vi "commander3.vi"() -> ()   [LabVIEW 2012]
uses:
  G_SEN.vi
  G_VEH.vi
  G_LCM.vi
  G_PATH.vi
  G_NAV.vi
  G_DATA.vi
  <vilib>/Analysis/Matrix/Datatypes/RealMatrix.ctl
  <vilib>/Analysis/Matrix/NI_Matrix.lvlib
panel:
  in  "x 2":dbl
  in  "mobileye":bool
  out "LCM Recv Data":string
  out "GPS DATA 2":T1={"type"="None", "x_lcc"=-59.06772232055664, "y_lcc"=-26.082616806030273, "latdev"=0.0, "londev"=0.0, "sats"=0, "gps_l1_ranges"=0, "gps_l1_mask_ranges"=0, "gps_l2_mask_ranges"=0, "Heading"=89.78975677490234, "lon"=0.0, "lat"=0.0, "time"="None", "hgps"=89.78975677490234, "lag"=89.78975677490234, "MAP"="None"} {"lag" format="%#_5g"; "hgps" format="%#_5g"; "lat" format="%#_11g"; "lon" format="%#_11g"; "Heading" format="%#_5g"; "latdev" format="%#_4g"; "londev" format="%#_4g"}
  in  "LCM":bool
  in  "obs":bool
  in  "x":dbl
  in  "log":bool
  in  "y":dbl min=-1.0 max=10.0 step=0.1
  out "timmer 2":u32
  out "timmer":u32
  out "Speed limit":dbl=8.0
  out "collision":bool
  out "Mission":i32=9
  in  "Load WPT":bool
  in  "Max. Vel.":dbl=20.0
  in  "RESET PATH":bool
  out "col":i16(graph)
  out "stop":bool
  in  "Reverse":bool
  in  "STOP":bool
  out "Waveform Chart 4":cluster{"auto":i16, "run":i16}(graph)={"auto"=1, "run"=0}
  out "Waveform Chart 3":T2(graph)={"Steer_input"=10.50986504720403, "Steer_output"=3.6, "handle"=10.50986504720403}
  out "Waveform Chart 2":T3(graph)={"VS_des"=4.606086314285715, "VS_can"=8.738, "VS_des"=5.0237113142857135}
  out "Heading":cluster{"Heading":dbl, "hgps":dbl}(graph)={"Heading"=269.76568785604456, "hgps"=270.2149981902155}
  out "XY Graph 2":cluster{"Y":dbl[], "Y":dbl[]}[](graph)=[{"Y"=[-241.57278442382812], "Y"=[-497.6172790527344]}, {"Y"=array[297 elements], "Y"=array[297 elements]}, {"Y"=array[297 elements], "Y"=array[297 elements]}, {"Y"=[-96.81030887093378], "Y"=[-438.1146154201037]}]
  out "Gauge":cluster{dbl, dbl, dbl}(knob)={4.606086314285715, 8.738, 5.0237113142857135} scale=-20.0..140.0
  out "Meter":cluster{dbl, dbl, dbl}(knob)={10.50986504720403, 3.6, 10.50986504720403} scale=-550.0..550.0
  out "XY Graph":cluster{"Y":dbl[], "Y":dbl[]}[](graph)=[{"Y"=[0.0], "Y"=[1000.0]}, {"Y"=[], "Y"=[]}, {"Y"=[], "Y"=[]}, {"Y"=[55.79381017995934], "Y"=[-143.41137512848826]}, {"Y"=[1.8243630881955273], "Y"=[-0.6091599202647308]}, {"Y"=[60.825233010671326, 56.37330625127248, 55.349089235151354, 59.801015994550255, 60.825233010671326], "Y"=[-144.72018116547483, -142.44414335187238, -144.44751039360185, -146.72354820720435, -144.72018116547483]}, {"Y"=[0.0, 2.210107140854234e-06, 8.840428449730098e-06, 1.9890964154001267e-05, 3.536171391260723e-05, 5.5252677611861145e-05, 7.956385525176302e-05, 0.00010829524660493917, 0.00014144685155770276, 0.0001790186695416196, 0.00022101070067037654, 0.00026742294460291305, 0.00031825540077079495, 0.00037350806894664856, 0.0004331809489031002, 0.0004972740399580289, 0.0005657873416566872, 0.0006387208537717015, 0.0007160745756209508, 0.0007978485066360008, 0.0008840426462484174, 0.0009746569938897665, 0.0010696915488779268, 0.0011691463105307776, 0.0012730212781661976, 0.001381316451102066, 0.0014940318285425747, 0.0016111674095782291, 0.0017327231935269083, 0.0018586991794791174, 0.001989095366525362, 0.00212391175364246, 0.002263148340148291, 0.0024068051247922995, 0.002554882106551304, 0.0027073792846294964, 0.002864296657776322, 0.003025634224741225, 0.003191391984614711, 0.0033615699362599116, 0.003536168078198898, 0.0037151864094084885, 0.003898624928524441, 0.004086483634296201, 0.004278762525359525, 0.004475461600350172, 0.0046765808579039, 0.004882120296656467, 0.0050920799150162566, 0.00530645971150534, 0.005525259684645789, 0.005748479832959674, 0.005976120154741693, 0.006208180648513917, 0.006444661312457356, 0.006685562145094082, 0.006930883144491418, 0.007180624309171435, 0.007434785636974084, 0.007693367126535122, 0.007956368775921874, 0.008223790583087975, 0.008495632546100751, 0.008771894663368585, 0.009052576932504053, 0.00933767935191554, 0.009627201919329309, 0.009921144632812684, 0.010219507490205615, 0.010522290489461739, 0.010829493628421005, 0.011141116904923365, 0.011457160316581394, 0.011777623861462416, 0.012102507536951634, 0.012431811341116372, 0.012765535271228146, 0.013103679325240591, 0.0134462435006526, 0.013793227794963059, 0.014144632205784546, 0.014500456730615952, 0.014860701366956164, 0.015225366112190386, 0.015594450963703821, 0.015967955919109045, 0.0163458809754502, 0.016728226130226176, 0.017114991380822175, 0.017506176724168654, 0.0179017821577645, 0.018301807678767545, 0.018706253284335617, 0.019115118971512857, 0.019528404737457095, 0.01994611057932616, 0.02036823649393682, 0.02079478247856059, 0.021225748530014243, 0.02166113464522823, 0.022100940821246695], "Y"=[0.0, 0.05249999993797367, 0.10499999950378934, 0.15749999832528905, 0.2099999960303148, 0.26249999224670867, 0.31499998660231265, 0.3674999787249688, 0.41999996824251923, 0.472499954782806, 0.5249999379736712, 0.577499917442957, 0.6299998928185055, 0.682499863728159, 0.7349998297997596, 0.7874997906611497, 0.8399997459401715, 0.8924996952646672, 0.9449996382624795, 0.9974995745614504, 1.0499995037894228, 1.1024994255742389, 1.1549993395437415, 1.2074992453257731, 1.2599991425481762, 1.3124990308387938, 1.3649989098254687, 1.4174987791360436, 1.4699986383983614, 1.5224984872402658, 1.574998325289599, 1.6274981521742047, 1.6799979675219257, 1.7324977709606055, 1.784997562118088, 1.837497340622216, 1.8899971061008334, 1.9424968581817836, 1.994996596492911, 2.047496320662059, 2.099996030317072, 2.152495725085793, 2.204995404596067, 2.2574950684757384, 2.309994716352652, 2.3624943478546507, 2.414993962609581, 2.467493560245286, 2.519993140389611, 2.5724927026704023, 2.6249922467155042, 2.6774917721527607, 2.7299912786100196, 2.7824907657151243, 2.834990233095921, 2.887489680380256, 2.939989107195975, 2.9924885131709242, 3.0449878979329497, 3.0974872611098974, 3.1499866023296144, 3.2024859212199472, 3.2549852174087435, 3.3074844905238483, 3.3599837401931105, 3.412482966044377, 3.464982167705495, 3.5174813448043127, 3.5699804969686775, 3.6224796238264374, 3.6749787250054404, 3.7274778001335362, 3.7799768488385714, 3.8324758707483966, 3.884974865490859, 3.9374738326938097, 3.989972771985096, 4.042471682992569, 4.094970565344078, 4.147469418667473, 4.199968242590603, 4.2524670367413195, 4.304965800747474, 4.3574645342369145, 4.409963236837495, 4.4624619081770645, 4.514960547883476, 4.567459155584579, 4.6199577309082285, 4.672456273482274, 4.724954782934569, 4.777453258892966, 4.829951700985317, 4.882450108839476, 4.934948482083297, 4.987446820344632, 5.039945123251335, 5.09244339043126, 5.144941621512262, 5.197439816122197, 5.249937973888915]}, {"Y"=[55.85492946607054, 56.300112183962334, 56.74529490185413, 57.19047761974598, 57.635660337637766, 58.08084305552956, 58.52602577342136, 58.97120849131315, 59.416391209205, 59.8615739270968, 60.306756644988596, 60.75193936288038, 61.197122080772175, 61.64230479866403, 62.087487516555825, 62.532670234447615, 62.97785295233941, 63.423035670231265, 63.86821838812306, 64.31340110601485, 64.75858382390665, 65.20376654179844, 65.64894925969023, 66.09413197758208, 66.53931469547388, 66.98449741336567, 67.42968013125746, 67.87486284914931, 68.3200455670411, 68.7652282849329, 69.2104110028247, 69.65559372071655, 70.10077643860835, 70.54595915650015, 70.99114187439193, 71.43632459228371, 71.88150731017556, 72.32669002806736, 72.77187274595916, 73.21705546385095], "Y"=[-143.26925304077835, -143.49687629901547, -143.72449955725253, -143.95212281548962, -144.17974607372668, -144.40736933196374, -144.63499259020085, -144.8626158484379, -145.090239106675, -145.3178623649121, -145.54548562314918, -145.7731088813862, -146.00073213962332, -146.22835539786038, -146.45597865609744, -146.68360191433456, -146.91122517257162, -147.1388484308087, -147.36647168904577, -147.59409494728285, -147.82171820551994, -148.04934146375703, -148.27696472199406, -148.50458798023115, -148.73221123846827, -148.9598344967053, -149.18745775494241, -149.4150810131795, -149.64270427141656, -149.87032752965362, -150.09795078789074, -150.3255740461278, -150.55319730436486, -150.78082056260195, -151.00844382083903, -151.23606707907612, -151.46369033731318, -151.6913135955503, -151.91893685378736, -152.14656011202442]}, {"Y"=[46.95734422441421, 47.0463827596022, 47.13542129479015, 47.224459829978144, 47.31349836516614, 47.40253690035408, 47.49157543554208, 47.58061397073008, 47.669652505918016, 47.75869104110601, 47.84772957629395, 47.936768111481946, 48.02580664666995, 48.11484518185789, 48.20388371704588, 48.292922252233886, 48.381960787421825, 48.47099932260982, 48.56003785779782, 48.64907639298576, 48.73811492817376, 48.827153463361746, 48.91619199854969, 49.00523053373769, 49.09426906892568, 49.18330760411363, 49.272346139301625, 49.361384674489564, 49.45042320967757, 49.53946174486556, 49.6285002800535, 49.717538815241504, 49.8065773504295, 49.89561588561743, 49.984654420805434, 50.07369295599343, 50.16273149118137, 50.251770026369364, 50.34080856155737, 50.429847096745306, 50.5188856319333, 50.607924167121304, 50.69696270230924, 50.78600123749724, 50.875039772685184, 50.96407830787318, 51.05311684306117, 51.142155378249115, 51.23119391343711, 51.320232448625106, 51.40927098381305, 51.49830951900105, 51.58734805418904, 51.67638658937698, 51.765425124564985, 51.85446365975298, 51.94350219494092, 52.03254073012892, 52.12157926531691, 52.21061780050485, 52.29965633569285, 52.38869487088079, 52.477733406068786, 52.56677194125679, 52.65581047644473, 52.74484901163272, 52.833887546820726, 52.922926082008665, 53.01196461719666, 53.10100315238466, 53.190041687572595, 53.27908022276059, 53.36811875794859, 53.45715729313653, 53.54619582832453, 53.635234363512524, 53.72427289870047, 53.813311433888465, 53.902349969076404, 53.99138850426441, 54.0804270394524, 54.16946557464034, 54.25850410982834, 54.34754264501633, 54.43658118020427, 54.525619715392274, 54.61465825058027, 54.70369678576821, 54.792735320956204, 54.88177385614421, 54.970812391332146, 55.05985092652014, 55.148889461708144, 55.23792799689608, 55.32696653208408, 55.41600506727202, 55.50504360246001, 55.59408213764801, 55.683120672835955, 55.77215920802395, 55.861197743211946, 55.95023627839994, 56.03927481358789, 56.12831334877588, 56.21735188396388, 56.306390419151825, 56.39542895433982, 56.48446748952781, 56.573506024715755, 56.66254455990375, 56.75158309509169, 56.84062163027969, 56.92966016546769, 57.01869870065563, 57.10773723584363, 57.196775771031625, 57.285814306219564, 57.37485284140757, 57.46389137659556, 57.552929911783494, 57.64196844697149, 57.73100698215949, 57.82004551734743, 57.90908405253543, 58.08716112291137, 58.176199658099364, 58.26523819328731, 58.354276728475305, 58.4433152636633, 58.53235379885125, 58.62139233403924, 58.71043086922723, 58.79946940441518, 58.88850793960317, 58.97754647479111, 59.06658500997911, 59.15562354516711, 59.24466208035505, 59.333700615543044, 59.42273915073105, 59.511777685918986, 59.60081622110698, 59.689854756294984, 59.778893291482916, 59.86793182667091, 59.956970361858914, 60.04600889704685, 60.13504743223485, 60.31312450261079, 60.402163037798786, 60.491201572986725, 60.58024010817473, 60.66927864336272, 60.75831717855066, 60.84735571373866, 60.93639424892665, 61.02543278411459, 61.114471319302595, 61.203509854490534, 61.29254838967853, 61.38158692486653, 61.47062546005447, 61.55966399524247, 61.64870253043047, 61.73774106561841, 61.826779600806404, 61.91581813599439, 62.00485667118234, 62.093895206370334, 62.18293374155833, 62.271972276746276, 62.36101081193427, 62.45004934712227, 62.53908788231021, 62.62812641749821, 62.71716495268615, 62.80620348787415, 62.895242023062146, 62.984280558250084, 63.07331909343808, 63.162357628626076, 63.251396163814015, 63.34043469900201, 63.42947323419001, 63.51851176937796, 63.60755030456595, 63.69658883975394, 63.78562737494189, 63.87466591012988, 63.96370444531783, 64.05274298050581, 64.14178151569382, 64.23082005088176, 64.31985858606976, 64.40889712125775, 64.4979356564457, 64.58697419163369, 64.76505126200964, 64.85408979719762, 64.94312833238557, 65.03216686757357, 65.12120540276156, 65.2102439379495, 65.29928247313751, 65.38832100832549, 65.47735954351344, 65.56639807870144, 65.65543661388938, 65.74447514907737, 65.83351368426537, 65.92255221945331, 66.0115907546413, 66.10062928982931, 66.18966782501724, 66.27870636020525, 66.36774489539324, 66.45678343058118, 66.54582196576918, 66.63486050095719, 66.72389903614511, 66.81293757133312, 66.9019761065211, 66.99101464170904, 67.08005317689705, 67.16909171208498, 67.25813024727299, 67.34716878246098, 67.43620731764892, 67.52524585283692, 67.61428438802493, 67.70332292321285, 67.79236145840086, 67.88139999358886, 67.97043852877678, 68.05947706396479, 68.14851559915279, 68.23755413434073, 68.32659266952872, 68.41563120471668, 68.50466973990466, 68.59370827509267, 68.6827468102806, 68.7717853454686, 68.8608238806566, 68.94986241584455, 69.03890095103253, 69.12793948622053, 69.21697802140848, 69.30601655659646, 69.39505509178447, 69.48409362697241, 69.5731321621604, 69.6621706973484, 69.75120923253635, 69.84024776772434, 69.92928630291229, 70.01832483810027, 70.10736337328828, 70.19640190847622, 70.2854404436642, 70.37447897885221, 70.46351751404015, 70.55255604922814, 70.64159458441614, 70.7306331196041, 70.81967165479207, 70.90871018998008, 70.99774872516802, 71.08678726035602, 71.17582579554401, 71.26486433073195, 71.35390286591995, 71.44294140110789, 71.5319799362959, 71.62101847148388, 71.71005700667183, 71.79909554185983, 71.88813407704782, 71.97717261223576, 72.06621114742377, 72.15524968261175, 72.2442882177997, 72.3333267529877, 72.42236528817568, 72.51140382336364, 72.60044235855163, 72.68948089373963, 72.77851942892757, 72.86755796411556, 72.9565964993035, 73.04563503449151, 73.13467356967949, 73.22371210486745, 73.31275064005544, 73.40178917524342, 73.49082771043138, 73.57986624561937], "Y"=[-138.89375124553214, -138.93927200180423, -138.98479275807625, -139.0303135143483, -139.07583427062036, -139.12135502689242, -139.16687578316444, -139.21239653943653, -139.25791729570855, -139.30343805198058, -139.34895880825266, -139.3944795645247, -139.44000032079677, -139.4855210770688, -139.53104183334085, -139.5765625896129, -139.62208334588496, -139.667604102157, -139.71312485842907, -139.7586456147011, -139.80416637097318, -139.8496871272452, -139.89520788351723, -139.9407286397893, -139.98624939606134, -140.0317701523334, -140.07729090860545, -140.1228116648775, -140.16833242114956, -140.2138531774216, -140.25937393369364, -140.30489468996572, -140.35041544623775, -140.39593620250977, -140.44145695878186, -140.48697771505388, -140.53249847132597, -140.578019227598, -140.62353998387005, -140.66906074014207, -140.71458149641416, -140.76010225268618, -140.80562300895826, -140.8511437652303, -140.89666452150234, -140.9421852777744, -140.98770603404643, -141.0332267903185, -141.07874754659053, -141.1242683028626, -141.16978905913462, -141.2153098154067, -141.26083057167872, -141.3063513279508, -141.35187208422283, -141.3973928404949, -141.44291359676694, -141.48843435303897, -141.53395510931105, -141.57947586558308, -141.62499662185516, -141.67051737812716, -141.71603813439924, -141.76155889067127, -141.80707964694335, -141.85260040321535, -141.89812115948743, -141.94364191575949, -141.9891626720315, -142.0346834283036, -142.08020418457562, -142.1257249408477, -142.1712456971197, -142.21676645339178, -142.2622872096638, -142.3078079659359, -142.3533287222079, -142.39884947847997, -142.44437023475203, -142.48989099102408, -142.53541174729614, -142.58093250356816, -142.62645325984025, -142.67197401611224, -142.71749477238433, -142.76301552865635, -142.80853628492844, -142.85405704120046, -142.89957779747255, -142.94509855374454, -142.99061931001663, -143.03614006628868, -143.0816608225607, -143.1271815788328, -143.17270233510482, -143.2182230913769, -143.2637438476489, -143.30926460392098, -143.354785360193, -143.4003061164651, -143.4458268727371, -143.4913476290092, -143.5368683852812, -143.58238914155328, -143.62790989782533, -143.67343065409736, -143.71895141036944, -143.76447216664147, -143.80999292291352, -143.85551367918555, -143.90103443545763, -143.94655519172966, -143.99207594800174, -144.03759670427374, -144.08311746054582, -144.12863821681785, -144.1741589730899, -144.21967972936199, -144.265200485634, -144.3107212419061, -144.3562419981781, -144.40176275445017, -144.4472835107222, -144.49280426699428, -144.58384577953836, -144.6293665358104, -144.67488729208247, -144.72040804835453, -144.76592880462653, -144.81144956089864, -144.85697031717064, -144.90249107344272, -144.94801182971474, -144.99353258598683, -145.03905334225882, -145.0845740985309, -145.13009485480293, -145.17561561107502, -145.22113636734704, -145.2666571236191, -145.31217787989118, -145.35769863616318, -145.40321939243526, -145.4487401487073, -145.49426090497937, -145.5397816612514, -145.58530241752348, -145.63082317379548, -145.7218646863396, -145.76738544261164, -145.8129061988837, -145.85842695515572, -145.90394771142783, -145.94946846769983, -145.9949892239719, -146.04050998024394, -146.08603073651602, -146.13155149278802, -146.1770722490601, -146.22259300533213, -146.2681137616042, -146.31363451787624, -146.3591552741483, -146.40467603042035, -146.45019678669237, -146.49571754296446, -146.54123829923648, -146.58675905550857, -146.6322798117806, -146.67780056805265, -146.72332132432467, -146.76884208059676, -146.81436283686878, -146.85988359314084, -146.9054043494129, -146.95092510568492, -146.99644586195703, -147.04196661822903, -147.0874873745011, -147.13300813077313, -147.17852888704522, -147.22404964331722, -147.2695703995893, -147.31509115586132, -147.3606119121334, -147.40613266840543, -147.4516534246775, -147.49717418094954, -147.54269493722157, -147.58821569349365, -147.63373644976568, -147.67925720603776, -147.72477796230976, -147.77029871858184, -147.81581947485387, -147.86134023112595, -147.90686098739798, -147.9979024999421, -148.0434232562141, -148.08894401248617, -148.13446476875822, -148.17998552503028, -148.22550628130233, -148.27102703757438, -148.3165477938464, -148.3620685501185, -148.40758930639052, -148.45311006266255, -148.49863081893463, -148.54415157520666, -148.58967233147874, -148.63519308775076, -148.6807138440228, -148.72623460029487, -148.77175535656693, -148.81727611283895, -148.86279686911104, -148.90831762538306, -148.95383838165512, -148.99935913792717, -149.0448798941992, -149.09040065047128, -149.1359214067433, -149.18144216301536, -149.22696291928742, -149.27248367555944, -149.31800443183153, -149.36352518810358, -149.4090459443756, -149.4545667006477, -149.50008745691972, -149.54560821319174, -149.59112896946382, -149.63664972573585, -149.68217048200793, -149.72769123827996, -149.77321199455199, -149.81873275082407, -149.86425350709612, -149.90977426336815, -149.95529501964023, -150.00081577591226, -150.0463365321843, -150.09185728845637, -150.1373780447284, -150.18289880100048, -150.2284195572725, -150.27394031354456, -150.3194610698166, -150.36498182608864, -150.4105025823607, -150.45602333863278, -150.5015440949048, -150.54706485117688, -150.5925856074489, -150.63810636372094, -150.68362711999302, -150.72914787626505, -150.7746686325371, -150.82018938880915, -150.86571014508118, -150.91123090135326, -150.9567516576253, -151.00227241389734, -151.04779317016943, -151.09331392644145, -151.13883468271348, -151.18435543898556, -151.2298761952576, -151.27539695152967, -151.3209177078017, -151.36643846407375, -151.4119592203458, -151.45747997661783, -151.5030007328899, -151.54852148916194, -151.594042245434, -151.63956300170608, -151.6850837579781, -151.73060451425013, -151.77612527052221, -151.82164602679424, -151.8671667830663, -151.91268753933835, -151.95820829561038, -152.00372905188246, -152.04924980815449, -152.09477056442654, -152.14029132069862, -152.18581207697065, -152.23133283324267, -152.27685358951476, -152.32237434578678, -152.36789510205887, -152.4134158583309, -152.45893661460295, -152.504457370875]}, {"Y"=[], "Y"=[]}, {"Y"=[], "Y"=[]}, {"Y"=[], "Y"=[]}, {"Y"=[-16.5, -15.25, -15.0, -13.5, -13.25, -13.25, -13.25, -13.0, -13.0, -12.75, -12.75, -12.75, -12.75, -12.75, -12.75, -12.75, -12.5, -12.5, -12.5, -12.5, -12.5, -12.5, -12.25, -12.25, -12.25, -12.25, -12.25, -12.25, -12.0, -12.0, -12.0, -11.75, -11.75, -11.75, -11.5, -11.5, -11.5, -11.5, -11.5, -11.25, -10.75, -10.75, -10.5, -10.5, -10.25, -10.25, -10.0, -10.0, -10.0, -10.0, -10.0, -9.75, -9.75, -9.75, -9.75, -9.75, -9.75, -9.75, -9.75, -9.75, -9.75, -9.5, -9.5, -9.5, -9.5, -9.5, -9.5, -9.5, -9.5, -9.5, -9.5, -9.5, -9.5, -9.5, -9.5, -9.5, -9.5, -9.5, -9.5, -9.5, -9.25, -9.25, -9.25, -9.25, -9.25, -9.25, -9.25, -9.25, -9.25, -9.25, -9.25, -9.25, -9.25, -9.25, -9.25, -9.25, -9.25, -9.25, -9.25, -9.25, -9.25, -9.25, -9.0, -9.0, -9.0, -9.0, -9.0, -9.0, -9.0, -9.0, -9.0, -9.0, -9.0, -9.0, -9.0, -9.0, -9.0, -9.0, -9.0, -9.0, -9.0, -9.0, -9.0, -9.0, -9.0, -9.0, -9.0, -9.0, -8.75, -8.75, -8.75, -8.75, -8.75, -8.75, -8.75, -8.75, -8.75, -8.75, -8.75, -8.75, -8.75, -8.75, -8.75, -8.75, -8.75, -8.75, -8.75, -8.75, -8.75, -8.75, -8.75, -8.75, -8.75, -8.75, -8.75, -8.75, -8.75, -8.75, -8.75, -8.75, -8.75, -8.75, -8.75, -8.75, -8.75, -8.5, -8.5, -8.5, -8.5, -8.5, -8.5, -8.5, -8.5, -8.5, -8.5, -8.5, -8.5, -8.5, -8.5, -8.5, -8.5, -8.5, -8.5, -8.5, -8.5, -8.5, -8.5, -8.5, -8.5, -8.5, -8.5, -8.5, -8.5, -8.5, -8.5, -8.5, -8.5, -8.5, -8.5, -8.5, -8.5, -8.25, -8.25, -8.25, -8.25, -8.25, -8.25, -8.25, -8.25, -8.25, -8.25, -8.25, -8.25, -8.25, -8.25, -8.25, -8.25, -8.25, -8.25, -8.25, -8.25, -8.25, -8.25, -8.25, -8.25, -8.25, -8.25, -8.25, -8.25, -8.25, -8.25, -8.25, -8.25, -8.25, -8.0, -8.0, -8.0, -8.0, -8.0, -8.0, -8.0, -8.0, -8.0, -8.0, -8.0, -8.0, -8.0, -8.0, -8.0, -8.0, -8.0, -8.0, -8.0, -8.0, -8.0, -8.0, -8.0, -8.0, -8.0, -7.75, -7.75, -7.75, -7.75, -7.75, -7.75, -7.75, -7.75, -7.75, -7.75, -7.75, -7.75, -7.75, -7.75, -7.75, -7.75, -7.75, -7.75, -7.75, -7.75, -7.75, -7.75, -7.75, -7.75, -7.75, -7.75, -7.5, -7.5, -7.5, -7.5, -7.5, -7.5, -7.5, -7.5, -7.5, -7.5, -7.5, -7.5, -7.5, -7.5, -7.5, -7.5, -7.5, -7.5, -7.5, -7.5, -7.5, -7.5, -7.5, -7.5, -7.5, -7.25, -7.25, -7.25, -7.25, -7.25, -7.25, -7.25, -7.25, -7.25, -7.25, -7.25, -7.25, -7.25, -7.25, -7.25, -7.25, -7.25, -7.25, -7.25, -7.25, -7.25, -7.25, -7.25, -7.0, -7.0, -7.0, -7.0, -7.0, -7.0, -7.0, -7.0, -7.0, -7.0, -7.0, -7.0, -7.0, -7.0, -7.0, -7.0, -7.0, -7.0, -7.0, -6.75, -6.75, -6.75, -6.75, -6.75, -6.75, -6.75, -6.75, -6.75, -6.75, -6.75, -6.75, -6.75, -6.75, -6.75, -6.75, -6.75, -6.75, -6.75, -6.75, -6.75, -6.75, -6.75, -6.5, -6.5, -6.5, -6.5, -6.5, -6.5, -6.5, -6.5, -6.5, -6.5, -6.5, -6.5, -6.5, -6.5, -6.5, -6.5, -6.5, -6.5, -6.5, -6.5, -6.5, -6.5, -6.5, -6.5, -6.5, -6.5, -6.5, -6.5, -6.5, -6.5, -6.25, -6.25, -6.25, -6.25, -6.25, -6.25, -6.25, -6.25, -6.25, -6.25, -6.25, -6.25, -6.25, -6.25, -6.25, -6.25, -6.25, -6.0, -6.0, -6.0, -6.0, -6.0, -6.0, -6.0, -6.0, -6.0, -6.0, -6.0, -5.75, -5.75, -5.75, -5.75, -5.75, -5.75, -5.75, -5.75, -5.75, -5.75, -5.5, -5.25, -5.0, -4.75, -4.5, -4.5, -4.25, -4.25, -4.0, -4.0, -3.75, -3.75, -3.5, -3.5, -3.25, -3.25, -3.25, -3.25, -3.0, -3.0, 2.0, 2.0, 2.0, 2.0, 2.0, 2.0, 2.0, 2.25, 2.25, 2.25, 2.25, 2.25, 2.25, 2.25, 2.25, 2.25, 2.25, 2.25, 2.25, 2.25, 2.25, 2.25, 2.25, 2.25, 2.25, 2.25, 2.25, 2.25, 2.25, 2.5, 2.5, 2.5, 2.5, 2.5, 2.5, 2.5, 2.5, 2.5, 2.5, 2.5, 2.5, 2.5, 2.5, 2.5, 2.5, 2.5, 2.5, 2.5, 2.5, 2.5, 2.5, 2.5, 2.5, 2.5, 2.5, 2.5, 2.5, 2.5, 2.5, 2.5, 2.5, 2.5, 2.5, 2.5, 2.5, 2.5, 2.5, 2.5, 2.5, 2.5, 2.5, 2.75, 2.75, 2.75, 2.75, 2.75, 2.75, 2.75, 2.75, 2.75, 2.75, 2.75, 2.75, 2.75, 2.75, 2.75, 2.75, 2.75, 2.75, 2.75, 2.75, 2.75, 2.75, 2.75, 2.75, 2.75, 2.75, 2.75, 2.75, 2.75, 2.75, 2.75, 2.75, 2.75, 2.75, 2.75, 2.75, 2.75, 2.75, 2.75, 2.75, 2.75, 2.75, 2.75, 2.75, 2.75, 2.75, 2.75, 2.75, 2.75, 2.75, 3.0, 3.0, 3.0, 3.0, 3.0, 3.0, 3.0, 3.0, 3.0, 3.0, 3.0, 3.0, 3.0, 3.0, 3.0, 3.0, 3.0, 3.0, 3.0, 3.0, 3.0, 3.0, 3.0, 3.0, 3.0, 3.0, 3.0, 3.0, 3.0, 3.0, 3.0, 3.0, 3.0, 3.0, 3.0, 3.0, 3.0, 3.0, 3.0, 3.0, 3.0, 3.0, 3.0, 3.0, 3.0, 3.0, 3.0, 3.25, 3.25, 3.25, 3.25, 3.25, 3.25, 3.25, 3.25, 3.25, 3.25, 3.25, 3.25, 3.25, 3.25, 3.25, 3.25, 3.25, 3.25, 3.25, 3.25, 3.25, 3.25, 3.25, 3.25, 3.25, 3.25, 3.25, 3.25, 3.25, 3.25, 3.25, 3.25, 3.25, 3.25, 3.25, 3.25, 3.25, 3.25, 3.25, 3.25, 3.25, 3.25, 3.25, 3.25, 3.25, 3.25, 3.25, 3.25, 3.25, 3.25, 3.25, 3.25, 3.25, 3.5, 3.5, 3.5, 3.5, 3.5, 3.5, 3.5, 3.5, 3.5, 3.5, 3.5, 3.5, 3.5, 3.5, 3.5, 3.5, 3.5, 3.5, 3.5, 3.5, 3.5, 3.5, 3.5, 3.5, 3.5, 3.5, 3.5, 3.5, 3.5, 3.5, 3.5, 3.5, 3.5, 3.5, 3.5, 3.5, 3.5, 3.5, 3.5, 3.5, 3.5, 3.5, 3.5, 3.5, 3.5, 3.5, 3.5, 3.5, 3.5, 3.5, 3.5, 3.5, 3.5, 3.5, 3.5, 3.5, 3.5, 3.75, 3.75, 3.75, 3.75, 3.75, 3.75, 3.75, 3.75, 3.75, 3.75, 3.75, 3.75, 3.75, 3.75, 3.75, 3.75, 3.75, 3.75, 3.75, 3.75, 3.75, 3.75, 3.75, 3.75, 3.75, 3.75, 3.75, 3.75, 3.75, 3.75, 3.75, 3.75, 3.75, 3.75, 3.75, 3.75, 3.75, 4.0, 4.0, 4.0, 4.0, 4.0, 4.0, 4.0, 4.0, 4.0, 4.0, 4.0, 4.0, 4.0, 4.0, 4.0, 4.0, 4.0, 4.0, 4.0, 4.0, 4.0, 4.0, 4.0, 4.0, 4.0, 4.0, 4.0, 4.0, 4.0, 4.0, 4.0, 4.0, 4.0, 4.0, 4.0, 4.0, 4.25, 4.25, 4.25, 4.25, 4.25, 4.25, 4.25, 4.25, 4.25, 4.25, 4.25, 4.25, 4.25, 4.25, 4.25, 4.25, 4.25, 4.25, 4.25, 4.25, 4.25, 4.25, 4.25, 4.25, 4.25, 4.25, 4.25, 4.25, 4.25, 4.25, 4.25, 4.25, 4.25, 4.25, 4.25, 4.25, 4.25, 4.25, 4.25, 4.25, 4.25, 4.25, 4.25, 4.5, 4.5, 4.5, 4.5, 4.5, 4.5, 4.5, 4.5, 4.5, 4.5, 4.5, 4.5, 4.5, 4.5, 4.5, 4.5, 4.5, 4.5, 4.5, 4.5, 4.5, 4.5, 4.5, 4.5, 4.5, 4.5, 4.5, 4.75, 4.75, 4.75, 4.75, 4.75, 4.75, 4.75, 4.75, 4.75, 4.75, 4.75, 4.75, 4.75, 4.75, 4.75, 4.75, 4.75, 4.75, 4.75, 4.75, 4.75, 4.75, 4.75, 4.75, 4.75, 4.75, 4.75, 4.75, 4.75, 5.0, 5.0, 5.0, 5.0, 5.0, 5.0, 5.0, 5.0, 5.0, 5.0, 5.0, 5.0, 5.0, 5.0, 5.0, 5.0, 5.0, 5.0, 5.0, 5.0, 5.0, 5.25, 5.25, 5.25, 5.25, 5.25, 5.25, 5.25, 5.25, 5.25, 5.25, 5.25, 5.25, 5.25, 5.25, 5.5, 5.5, 5.5, 5.5, 5.5, 5.5, 5.5, 5.5, 5.5, 5.5, 5.5, 5.5, 5.75, 5.75, 5.75, 5.75, 5.75, 5.75, 5.75, 5.75, 5.75, 5.75, 5.75, 5.75, 5.75, 5.75, 5.75, 5.75, 5.75, 6.0, 6.0, 6.0, 6.0, 6.0, 6.0, 6.0, 6.0, 6.0, 6.0, 6.0, 6.25, 6.25, 6.25, 6.25, 6.25, 6.25, 6.25, 6.25, 6.5, 6.5, 6.5, 6.5, 6.5, 6.5, 6.5, 6.5, 6.5, 6.75, 6.75, 6.75, 6.75, 7.0, 7.0, 7.0, 7.25, 7.25, 7.25, 7.25, 7.25, 7.25, 7.25, 7.5, 7.5, 8.0, 8.0, 8.0, 8.0, 8.0, 8.25, 8.25, 8.5, 8.5, 8.5, 8.75, 8.75, 8.75, 8.75, 8.75, 9.0, 9.0, 9.0, 9.0, 9.0, 9.0, 9.25, 9.25, 9.25, 9.25, 9.25, 9.25, 9.5, 9.5, 9.5, 9.5, 9.5, 9.5, 9.75, 9.75, 9.75, 10.0, 10.0, 10.0, 10.0, 10.25, 10.25, 10.5, 10.5, 10.5, 10.75, 10.75, 10.75, 10.75, 11.0, 11.0, 11.0, 11.0, 11.0, 11.25, 11.25, 11.25, 11.25, 11.25, 11.25, 11.25, 11.25, 11.25, 11.25, 11.5, 11.5, 11.5, 11.5, 11.5, 11.5, 11.5, 11.5, 11.5, 11.5, 11.5, 11.5, 11.5, 11.5, 11.5, 11.75, 11.75, 11.75, 11.75, 11.75, 11.75, 11.75, 11.75, 11.75, 11.75, 11.75, 11.75, 11.75, 11.75, 11.75, 11.75, 11.75, 11.75, 11.75, 11.75, 12.0, 12.0, 12.0, 12.0, 12.0, 12.0, 12.0, 12.0, 12.0, 12.0, 12.0, 12.0, 12.0, 12.0, 12.0, 12.0, 12.0, 12.0, 12.0, 12.0, 12.0, 12.0, 12.0, 12.0, 12.0, 12.0, 12.0, 12.25, 12.25, 12.25, 12.25, 12.25, 12.25, 12.25, 12.25, 12.25, 12.25, 12.25, 12.25, 12.25, 12.25, 12.25, 12.25, 12.5, 12.5, 12.5, 12.5, 12.5, 12.5, 12.5, 12.5, 12.5, 12.5, 12.5, 12.5, 12.5, 12.75, 12.75, 12.75, 12.75, 12.75, 12.75, 12.75, 12.75, 12.75, 12.75, 13.0, 13.0, 13.0, 13.0, 13.0, 13.0, 13.0, 13.0, 13.0, 13.0, 13.0, 13.0, 13.0, 13.0, 13.0, 13.0, 13.0, 13.0, 13.0, 13.0, 13.0, 13.0, 13.0, 13.25, 13.25, 13.25, 13.25, 13.25, 13.25, 13.25, 13.25, 13.25, 13.25, 13.25, 13.25, 13.25, 13.25, 13.25, 13.25, 13.25, 13.25, 13.25, 13.5, 13.5, 13.5, 13.5, 13.5, 13.5, 13.5, 13.5, 13.5, 13.5, 13.75, 13.75, 13.75, 13.75, 13.75, 13.75, 13.75, 13.75, 13.75, 14.0, 14.0, 14.0, 14.0, 14.5, 14.75, 15.5, 15.75, 16.0, 19.25, 19.25, 19.25, 19.5, 19.5, 19.75, 22.25, 22.25, 22.25, 22.5, 22.5, 22.5, 22.75, 22.75, 22.75, 22.75, 23.0, 23.0, 23.0, 23.25, 23.25, 23.25, 23.5, 23.5, 23.5, 23.5, 23.5, 23.5, 23.75, 23.75, 23.75, 23.75, 23.75, 23.75, 23.75, 23.75, 23.75, 23.75, 23.75, 24.0, 24.0, 24.0, 24.0, 24.0, 24.0, 24.0, 24.25, 24.25, 24.5], "Y"=[46.5, 46.5, 46.5, 2.75, 0.5, 2.75, 17.0, 0.75, 17.25, -6.5, -2.25, -1.75, 0.5, 0.75, 1.0, 3.75, -6.5, 0.75, 4.0, 4.25, 17.25, 21.5, -6.75, -6.5, -1.75, 17.25, 21.5, 22.25, -6.75, 21.75, 22.0, -6.5, 11.25, 22.0, 10.5, 10.75, 11.0, 11.5, 11.75, -6.0, 3.75, 8.25, -1.0, 8.25, -1.25, -1.0, -7.0, -1.25, 2.75, 3.0, 3.5, -10.75, -10.5, -10.0, -9.5, -9.25, -8.25, -6.75, -1.25, 3.0, 3.25, -20.5, -15.5, -15.25, -14.75, -10.5, -10.25, -10.0, -9.75, -9.25, -9.0, -8.75, -8.25, -8.0, -7.75, -7.5, -1.0, 0.5, 1.5, 2.75, -20.25, -18.25, -17.75, -17.5, -17.0, -15.75, -15.5, -10.75, -10.25, -9.5, -9.0, -8.75, -8.25, -8.0, -7.75, 0.75, 1.0, 1.25, 2.25, 3.5, 7.25, 7.5, -19.0, -17.5, -17.25, -10.5, -10.25, -10.0, -9.25, -9.0, -8.75, -8.25, -8.0, -7.25, -7.0, -6.75, -4.75, -4.5, -4.25, 0.75, 1.0, 1.25, 1.75, 2.25, 2.5, 2.75, 3.5, 7.5, -17.5, -12.75, -12.0, -11.75, -10.5, -9.75, -9.5, -9.25, -9.0, -8.75, -8.5, -8.25, -8.0, -7.75, -7.5, -7.0, -6.75, -4.75, -4.5, -3.75, -3.25, -3.0, -1.5, -0.5, -0.25, 0.0, 0.25, 1.75, 2.5, 2.75, 4.25, 4.75, 5.5, 5.75, 6.25, 7.5, 7.75, -13.25, -13.0, -12.75, -12.0, -11.75, -8.25, -8.0, -7.0, -6.75, -5.5, -5.0, -4.75, -4.5, -4.0, -3.75, -3.25, -3.0, -2.75, -2.0, -1.75, -1.5, -1.0, -0.5, -0.25, 0.0, 0.25, 0.5, 0.75, 1.75, 2.0, 4.0, 4.25, 4.75, 5.75, 6.0, 6.25, -17.5, -12.75, -12.0, -11.5, -10.25, -8.25, -8.0, -7.75, -5.5, -4.75, -4.0, -3.75, -3.5, -3.25, -3.0, -2.75, -2.5, -2.25, -2.0, -1.75, -1.5, -0.75, -0.5, -0.25, 0.0, 0.25, 0.5, 2.25, 4.5, 4.75, 5.75, 6.0, 6.25, -13.5, -13.25, -13.0, -7.75, -5.75, -5.5, -5.25, -5.0, -4.75, -4.5, -3.75, -3.5, -3.25, -2.25, -2.0, -1.75, -1.5, -1.25, -0.75, -0.5, -0.25, 0.0, 0.25, 0.5, 0.75, -13.25, -12.5, -6.0, -5.75, -5.25, -5.0, -4.75, -4.5, -4.25, -3.25, -2.5, -2.25, -2.0, -1.75, -1.5, -1.25, -0.75, -0.5, -0.25, 0.0, 0.25, 0.5, 4.0, 4.25, 7.75, 8.0, -14.0, -13.25, -13.0, -8.0, -5.25, -5.0, -4.75, -3.75, -3.0, -2.0, -1.75, -1.5, -1.25, -0.5, -0.25, 0.25, 0.5, 0.75, 1.0, 1.25, 1.5, 2.25, 2.5, 3.75, 9.25, -7.75, -7.25, -7.0, -6.75, -6.5, -6.25, -6.0, -5.75, -5.5, -5.25, -5.0, -3.5, -1.75, -1.5, -1.25, -0.5, -0.25, 1.0, 1.25, 1.75, 2.5, 5.75, 8.5, -9.0, -8.0, -7.75, -7.0, -6.75, -6.5, -5.5, -5.25, -5.0, -2.0, -1.75, 1.25, 1.5, 2.5, 4.0, 4.25, 4.5, 6.0, 8.5, -9.25, -9.0, -7.5, -7.25, -5.75, -5.5, -2.75, -2.5, -1.0, -0.75, -0.5, -0.25, 0.0, 1.0, 1.25, 1.75, 2.75, 3.0, 4.5, 4.75, 5.75, 6.0, 6.25, -20.0, -8.0, -7.5, -7.25, -4.5, -4.25, -3.25, -3.0, -2.75, -2.5, -1.25, -1.0, -0.75, -0.5, 2.25, 2.5, 2.75, 3.0, 3.25, 3.5, 3.75, 4.0, 4.25, 4.5, 4.75, 5.0, 5.25, 5.5, 5.75, 6.0, -20.25, -20.0, -14.0, -13.75, -8.0, -7.75, -7.25, -5.0, -4.75, -4.5, -3.5, -3.25, -3.0, -2.0, -1.75, -1.5, 3.0, -20.0, -14.0, -13.75, -8.0, -7.75, -7.5, -7.25, -5.0, -2.0, -1.75, -1.5, -20.5, -20.25, -14.25, -8.0, -7.75, -7.5, -2.0, -1.75, -1.5, 3.0, 3.0, 3.0, 3.0, 3.0, 3.0, 20.75, 3.0, 20.75, 3.0, 20.75, 3.0, 20.75, 3.0, 20.75, 3.0, 21.0, 22.0, 22.25, 3.0, 22.25, -8.25, -8.0, -7.25, -2.75, -2.5, -2.25, -2.0, -20.5, -14.5, -14.25, -8.5, -8.25, -8.0, -7.75, -7.25, -4.5, -4.0, -3.5, -3.25, -3.0, -2.5, -2.25, -2.0, -1.5, -1.25, -1.0, 4.75, 6.0, 6.25, -20.5, -20.25, -14.25, -8.25, -8.0, -7.75, -5.0, -4.5, -4.25, -4.0, -3.75, -3.5, -3.25, -3.0, -2.75, -2.5, -2.25, -2.0, -1.75, -1.5, -1.25, -1.0, -0.75, 0.75, 1.75, 2.0, 2.25, 2.5, 2.75, 3.0, 3.25, 3.5, 3.75, 4.0, 5.0, 5.25, 5.5, 5.75, 6.25, 6.5, 6.75, 7.0, -20.5, -20.25, -14.25, -8.25, -7.75, -4.75, -4.5, -4.25, -4.0, -3.75, -3.5, -3.25, -3.0, -2.75, -2.5, -2.0, -1.75, -1.5, -1.25, -1.0, -0.75, -0.5, 0.25, 0.5, 0.75, 1.0, 1.25, 1.5, 1.75, 2.0, 2.25, 2.5, 2.75, 3.25, 3.5, 3.75, 4.0, 4.25, 4.5, 4.75, 5.0, 5.25, 5.5, 5.75, 6.0, 6.25, 6.5, 6.75, 7.0, 7.25, -20.25, -7.75, -5.25, -4.5, -4.25, -4.0, -3.75, -3.5, -3.25, -2.75, -2.5, -2.25, -2.0, -1.75, -1.5, -1.25, -1.0, -0.75, -0.5, -0.25, 0.0, 0.25, 0.5, 0.75, 1.0, 1.25, 1.5, 1.75, 2.0, 2.25, 2.5, 2.75, 4.25, 4.5, 4.75, 5.0, 5.25, 5.5, 5.75, 6.0, 6.25, 6.5, 6.75, 7.0, 7.5, 9.5, 10.75, -20.5, -7.5, -6.75, -6.0, -5.75, -5.0, -4.75, -4.5, -4.25, -4.0, -3.25, -3.0, -2.75, -2.5, -2.0, -1.75, -1.5, -1.25, -1.0, -0.75, -0.5, -0.25, 0.0, 0.25, 0.5, 0.75, 1.0, 1.25, 1.5, 1.75, 2.0, 2.25, 2.5, 2.75, 3.0, 4.5, 4.75, 5.0, 5.25, 5.5, 5.75, 6.0, 6.25, 6.5, 6.75, 7.0, 7.25, 9.25, 9.5, 10.75, 11.0, 12.25, 12.75, -7.75, -7.5, -6.75, -6.5, -5.75, -5.5, -5.25, -4.75, -4.25, -4.0, -3.5, -3.0, -2.75, -2.25, -2.0, -1.75, -1.5, -1.25, -1.0, -0.75, -0.5, -0.25, 0.0, 0.25, 0.5, 0.75, 1.0, 1.25, 1.5, 1.75, 2.0, 2.25, 2.5, 2.75, 3.0, 4.75, 5.0, 5.25, 5.5, 5.75, 6.0, 6.5, 6.75, 7.0, 8.75, 9.0, 9.25, 10.25, 10.75, 11.0, 11.25, 12.25, 12.5, 12.75, 13.0, 13.25, 13.75, -8.75, -7.5, -6.5, -6.25, -5.5, -5.0, -4.75, -4.5, -4.25, -4.0, -2.25, -1.75, -1.5, -1.25, -1.0, -0.75, -0.5, -0.25, 0.0, 0.25, 0.5, 1.0, 1.25, 1.5, 1.75, 2.0, 2.25, 2.5, 2.75, 3.0, 3.25, 9.75, 11.0, 11.25, 12.25, 12.5, 13.0, -8.5, -7.5, -6.75, -6.5, -5.5, -5.25, -4.25, -4.0, -3.25, -3.0, -2.75, -2.5, -2.25, -1.75, -1.5, -1.25, -1.0, -0.75, -0.5, -0.25, 0.0, 0.25, 0.5, 0.75, 1.0, 1.25, 1.5, 1.75, 2.0, 2.25, 2.5, 2.75, 3.0, 12.5, 13.0, 13.25, -9.75, -9.5, -9.25, -8.75, -8.5, -8.25, -7.75, -7.5, -7.25, -7.0, -6.75, -6.5, -6.25, -6.0, -5.75, -5.0, -4.25, -3.0, -2.75, -2.5, -2.25, -1.75, -1.5, 0.0, 0.25, 0.5, 0.75, 1.0, 1.25, 1.5, 1.75, 2.0, 2.5, 2.75, 3.0, 3.25, 11.0, 11.25, 11.5, 12.0, 12.25, 12.5, 13.0, -10.0, -9.0, -8.75, -8.5, -8.25, -7.5, -7.25, -6.5, -6.0, -5.75, -4.5, -4.25, -4.0, -3.0, 0.25, 0.5, 0.75, 1.0, 2.5, 2.75, 3.0, 3.5, 11.5, 11.75, 12.0, 12.25, 12.75, -11.25, -10.75, -10.0, -9.5, -9.25, -9.0, -8.75, -8.0, -7.25, -7.0, -6.5, -6.25, -6.0, -5.75, -5.5, -4.75, -4.5, -4.25, -4.0, -3.75, 2.25, 2.5, 2.75, 3.0, 3.5, 6.75, 11.25, 11.5, 12.0, -12.25, -9.0, -8.75, -6.5, -6.25, -6.0, -5.75, -5.5, -5.25, -5.0, -4.75, -4.25, -4.0, -3.75, -3.5, 1.25, 2.5, 2.75, 3.25, 6.75, 12.0, -9.0, -8.75, -8.5, -7.0, -5.75, -5.5, -4.25, -3.5, -3.25, -3.0, -0.75, 2.0, 2.25, 12.0, -10.75, -9.0, -8.25, -3.25, -3.0, 2.0, 2.25, 2.5, 4.25, 5.75, 12.0, 13.0, -9.0, -3.5, 1.0, 1.25, 1.5, 1.75, 2.25, 2.5, 2.75, 3.25, 5.5, 5.75, 8.25, 8.5, 8.75, 9.0, 9.25, -9.0, -8.75, 1.5, 1.75, 3.25, 3.5, 5.5, 5.75, 6.25, 8.25, 9.0, -9.0, -8.75, 1.75, 3.25, 3.75, 5.75, 9.0, 9.5, -17.25, 1.5, 1.75, 3.25, 4.75, 5.5, 6.0, 6.25, 6.75, 4.5, 4.75, 5.5, 6.25, 4.5, 4.75, 5.75, 4.5, 6.25, 8.75, 9.0, 10.25, 10.5, 17.0, 4.0, 17.0, 1.5, 6.75, 10.75, 11.0, 17.5, 0.0, 17.5, 3.25, 17.25, 17.5, 0.25, 3.0, 3.25, 11.25, 11.5, -0.5, 6.75, 11.25, 11.5, 12.25, 35.5, -11.25, 12.0, 12.25, 12.75, 17.0, 35.5, -13.0, -12.25, -10.75, 12.0, 12.25, 17.0, 16.5, 16.75, 28.5, 16.25, 16.5, 28.25, 28.75, 28.0, 28.5, 2.25, 28.0, 28.25, 2.0, 2.5, 3.25, 8.0, 2.75, 3.25, 8.0, 8.25, 15.75, -7.75, -7.5, -5.25, -4.75, -2.25, 5.25, 8.0, 8.25, 15.25, 15.5, -9.25, -7.25, -4.75, -3.5, -3.0, -2.5, 2.5, 4.0, 4.25, 4.5, 4.75, 7.0, 7.75, 8.75, 9.0, -7.75, 1.0, 1.5, 2.25, 2.5, 2.75, 3.0, 3.25, 3.5, 3.75, 4.0, 4.25, 4.5, 4.75, 5.0, 5.25, 6.25, 8.0, 10.5, 28.75, -11.25, -7.25, 1.5, 1.75, 2.0, 2.25, 2.5, 2.75, 3.0, 3.25, 3.5, 3.75, 4.0, 4.25, 4.75, 5.0, 5.25, 5.5, 5.75, 6.0, 6.25, 6.5, 7.0, 7.25, 7.5, 7.75, 14.25, 1.75, 2.0, 2.5, 3.25, 3.75, 4.0, 5.75, 6.0, 6.25, 6.5, 6.75, 7.5, 9.25, 13.0, 13.25, 14.0, 1.75, 2.0, 2.5, 3.0, 3.25, 3.5, 6.0, 8.0, 8.25, 9.25, 10.25, 13.5, 13.75, -1.75, -1.5, -1.25, 3.25, 3.5, 4.0, 7.0, 8.0, 9.0, 13.0, -9.5, -5.0, -4.5, -4.25, -4.0, -3.75, -2.0, -1.75, -1.5, -1.25, -1.0, -0.75, -0.5, -0.25, 0.0, 0.25, 6.0, 7.5, 8.75, 9.5, 10.25, 12.25, 12.5, -5.5, -5.25, -5.0, -4.75, -4.5, -4.0, -3.75, -3.5, -2.0, -1.75, -1.0, -0.25, 0.25, 1.0, 1.25, 1.5, 7.5, 10.5, 10.75, -6.75, -6.5, -6.25, -6.0, -5.75, -5.5, 1.0, 1.25, 5.75, 10.5, -7.5, -7.25, -7.0, -6.75, -6.5, -3.5, -3.25, 1.25, 10.25, -7.0, -6.75, -3.5, 9.0, -4.0, -4.25, 17.25, 17.0, 17.0, 3.0, 3.25, 16.5, 16.5, 16.75, 3.0, 13.0, 13.25, 13.5, 13.75, 14.0, 14.25, 14.5, 14.75, 15.0, 15.25, 15.25, 15.5, 15.75, 16.0, 16.25, 16.5, 4.75, 5.0, 10.25, 16.75, 17.0, 17.25, 4.25, 4.5, 4.75, 5.0, 5.25, 5.5, 5.75, 6.0, 6.25, 6.5, 10.25, 4.25, 6.5, 6.75, 7.0, 7.25, 7.5, 7.75, 8.0, 10.0, 10.0]}, {"Y"=[-1.75], "Y"=[8.75]}, {"Y"=[-23.75, -23.5, -23.5, -22.0, -21.75, -17.5, -13.0, -13.0, -12.75, -12.5, -12.25, -11.5, -10.75, -10.75, -10.5, -10.5, -10.5, -10.5, -10.25, -10.25, -10.25, -10.0, -9.75, -9.5, -9.5, -9.5, -9.25, -9.25, -9.0, -9.0, -9.0, -9.0, -8.75, -8.75, -8.75, -8.75, -8.75, -8.75, -8.75, -8.75, -8.75, -8.5, -8.5, -8.5, -8.5, -8.5, -8.5, -8.5, -8.25, -8.25, -8.25, -8.25, -8.25, -8.25, -8.25, -8.25, -8.25, -8.25, -8.25, -8.0, -8.0, -8.0, -8.0, -7.75, -7.75, -7.75, -7.75, -7.75, -7.75, -7.75, -7.75, -7.75, -7.5, -7.5, -7.5, -7.5, -7.5, -7.5, -7.5, -7.5, -7.5, -7.5, -7.5, -7.5, -7.25, -7.25, -7.25, -7.25, -7.25, -7.25, -7.25, -7.25, -7.25, -7.25, -7.25, -7.25, -7.25, -7.25, -7.0, -7.0, -7.0, -7.0, -7.0, -7.0, -7.0, -7.0, -7.0, -7.0, -6.75, -6.75, -6.75, -6.75, -6.75, -6.75, -6.75, -6.75, -6.75, -6.75, -6.75, -6.5, -6.5, -6.5, -6.5, -6.5, -6.25, -6.25, -6.25, -6.25, -6.25, -6.25, -6.25, -6.25, -6.25, -6.25, -6.25, -6.25, -6.0, -6.0, -5.75, -5.75, -5.75, -5.75, -5.75, -5.75, -5.75, -5.75, -5.75, -5.75, -5.75, -5.75, -5.75, -5.75, -5.75, -2.25, -2.25, -2.25, -2.25, -2.25, -2.25, -2.25, -2.25, -2.25, -2.25, -2.25, -2.25, -2.25, -2.25, -2.25, -2.25, -2.25, -2.25, -2.0, -2.0, -2.0, -2.0, -2.0, -2.0, -2.0, -2.0, -2.0, -2.0, -2.0, -2.0, -2.0, -2.0, -2.0, -2.0, -2.0, -2.0, -2.0, -2.0, -2.0, -2.0, -2.0, -2.0, -1.75, -1.75, -1.75, -1.75, -1.75, -1.75, -1.75, -1.75, -1.75, -1.75, -1.75, -1.75, -1.75, -1.75, -1.75, -1.75, -1.75, -1.5, -1.5, -1.5, -1.5, -1.5, -1.5, -1.5, -1.5, -1.5, -1.5, -1.5, -1.5, -1.5, -1.25, -1.25, 1.75, 1.75, 1.75, 1.75, 1.75, 1.75, 1.75, 1.75, 1.75, 1.75, 1.75, 1.75, 1.75, 2.0, 2.0, 2.0, 2.0, 2.0, 2.0, 2.0, 2.0, 2.0, 2.0, 2.25, 2.25, 2.5, 2.5, 2.5, 2.5, 2.5, 2.5, 2.75, 2.75, 2.75, 2.75, 2.75, 2.75, 2.75, 2.75, 2.75, 3.0, 3.0, 3.0, 3.0, 3.0, 3.0, 3.0, 3.0, 3.25, 3.25, 3.25, 3.25, 3.25, 3.25, 3.25, 3.25, 3.5, 3.5, 3.5, 3.5, 3.5, 3.75, 4.0, 4.0, 4.0, 4.0, 4.25, 4.25, 4.25, 4.5, 4.5, 4.5, 4.5, 4.75, 4.75, 4.75, 5.0, 5.0, 5.5, 6.5, 7.0, 7.0, 7.25, 7.5, 7.5, 7.75, 7.75, 8.0, 8.25, 8.5, 8.75, 8.75, 10.5, 10.75, 11.0, 11.0, 11.0, 11.0, 11.0, 11.0, 11.25, 11.25, 11.25, 11.25, 11.25, 11.25, 11.25, 11.25, 11.5, 11.5, 11.5, 11.5, 11.5, 11.5, 11.5, 11.5, 11.5, 11.5, 11.5, 11.5, 11.75, 11.75, 11.75, 11.75, 11.75, 12.0, 12.0, 12.0, 12.0, 12.0, 12.0, 12.0, 12.25, 12.25, 12.5, 12.75, 13.5, 13.5, 13.5, 13.5, 13.5, -2.25, -2.25, -1.75], "Y"=[24.75, 24.75, 25.0, 24.75, 24.75, 15.25, 1.0, 4.5, 20.0, 19.75, 0.5, 14.25, 14.25, 14.5, 6.0, 14.5, 14.75, 15.5, 14.75, 15.0, 15.25, 9.5, 3.5, -3.0, 3.0, 3.25, 8.25, 16.75, 0.5, 1.5, 8.25, 12.25, 1.0, 1.25, 1.5, 2.0, 2.25, 6.0, 8.0, 8.5, 12.75, -11.5, -5.75, 1.0, 2.25, 3.0, 9.0, 12.75, -13.25, -11.0, -4.5, -1.25, 3.0, 3.25, 4.0, 6.5, 8.75, 9.0, 9.25, -15.0, 8.75, 9.0, 9.25, -13.5, -8.0, -6.25, -3.0, -2.75, 1.75, 2.0, 2.25, 9.75, -11.5, -4.5, -2.75, -1.0, -0.75, 0.0, 2.0, 2.75, 3.0, 7.0, 7.25, 7.5, -14.25, -11.5, -8.5, -8.0, -4.75, -4.25, -3.25, -3.0, -0.75, 0.25, 0.75, 2.75, 3.0, 7.75, -14.75, -14.5, -11.5, -8.25, -1.5, -1.25, 1.0, 8.0, 8.25, 10.5, -11.75, 0.25, 0.5, 0.75, 1.5, 2.0, 2.25, 2.5, 6.5, 6.75, 8.25, -19.0, 0.25, 0.5, 0.75, 6.25, -5.75, -2.5, -0.25, 0.0, 0.25, 0.5, 0.75, 1.0, 1.25, 1.5, 1.75, 2.0, 5.0, 6.25, -12.25, -10.0, -5.25, -4.25, -4.0, -3.0, -0.75, -0.5, -0.25, 2.0, 2.25, 2.5, 3.75, 4.0, 5.0, -3.25, -3.0, -2.5, -2.25, 3.0, 3.25, 3.5, 3.75, 4.0, 4.25, 4.5, 4.75, 5.0, 5.25, 5.5, 6.0, 6.5, 7.25, -12.75, -10.75, -9.25, -9.0, -8.0, -7.0, -6.25, -5.5, -5.0, -4.5, -4.0, -3.5, -3.25, -3.0, -2.75, -2.5, -2.25, 3.0, 3.25, 3.5, 3.75, 4.25, 4.5, 15.25, -15.5, -12.75, -10.75, 3.5, 3.75, 4.0, 4.25, 4.5, 4.75, 5.0, 5.25, 5.75, 6.25, 6.75, 7.25, 8.0, 15.25, -12.75, -10.75, -9.25, -8.0, -7.0, -6.25, -5.75, -5.25, -5.0, -4.5, -4.25, -3.75, -3.5, -15.75, -12.75, 3.25, 3.5, 3.75, 4.0, 4.25, 4.5, 4.75, 5.0, 5.25, 5.75, 6.25, 6.75, 7.25, -13.0, -4.5, -4.25, -3.75, 6.0, 6.25, 6.75, 7.25, 8.0, 8.75, 3.75, 10.0, 4.25, 4.5, 4.75, 6.0, 7.75, 11.25, -7.0, -6.0, -5.25, 7.5, 7.75, 8.5, 9.5, 9.75, 12.75, -12.5, -12.25, -6.75, -6.0, -5.75, 8.25, 8.5, 9.25, -10.5, -8.75, -8.5, 9.0, 10.25, 10.5, 12.5, 15.25, -15.5, -15.0, -10.5, -8.75, 10.5, -3.25, -12.5, -12.25, -10.0, -6.25, -8.0, -5.5, 2.25, -9.75, -8.0, -6.25, -4.75, -12.75, -5.25, -5.0, -12.5, 1.5, 1.5, 3.75, 1.25, 5.5, 5.5, 3.5, 5.75, 1.75, 3.5, 3.5, 8.0, 3.75, -1.5, 8.25, 3.5, 3.0, 2.5, 4.0, 4.25, 4.75, 5.25, 9.25, -5.5, -3.75, -2.0, 1.75, 3.25, 3.5, 8.5, 10.75, -7.5, -5.25, 1.25, 3.0, 3.25, 3.5, 8.0, 8.5, 9.5, 9.75, 10.25, 10.5, -7.5, -5.25, 1.75, 2.0, 7.5, -4.5, -4.25, -3.75, 6.75, 8.0, 13.75, 14.0, -3.5, 13.5, 12.25, 12.5, -0.75, -0.5, -0.25, 0.0, 0.25, 8.75, 12.75, 8.75]}, {"Y"=[0.85, 0.95, 0.95, 0.6, 0.6, 0.85, 0.85, -0.85, -0.85, -0.95, -0.95, -0.6, -0.6, -0.85, -0.6, -0.6, -0.85, -0.85, 0.85, 0.85], "Y"=[-0.6, -0.6, -1.4, -1.4, -0.6, -0.6, 2.4, 2.4, -0.6, -0.6, -1.4, -1.4, -0.6, -0.6, -0.6, -1.4, -1.4, -1.6, -1.6, -1.4]}]
  in  "Make WPT":bool
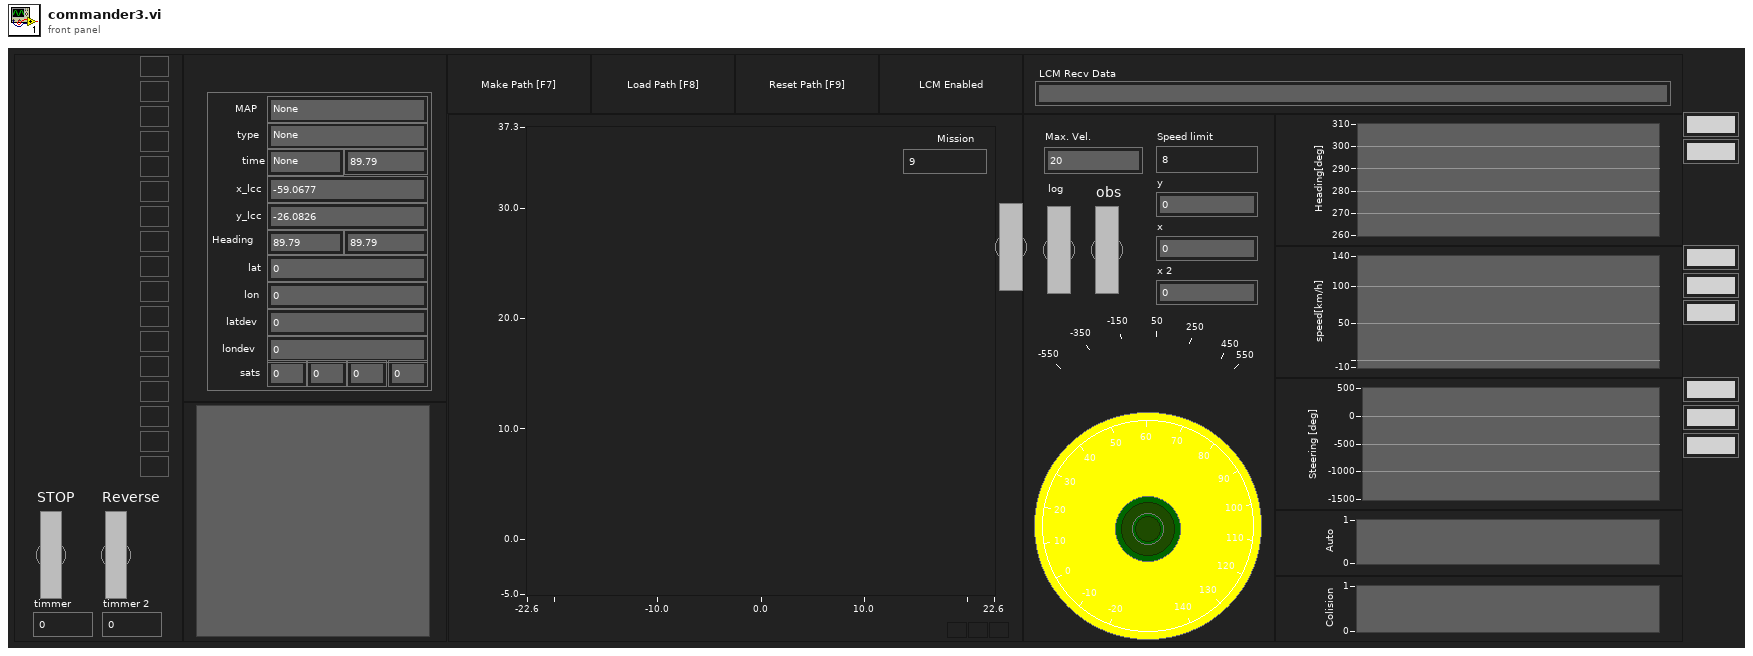
[diagram p1: front panel]
types:
  T1 = cluster{"type":string, "x_lcc":dbl, "y_lcc":dbl, "latdev":sgl, "londev":sgl, "sats":u8, "gps_l1_ranges":u8, "gps_l1_mask_ranges":u8, "gps_l2_mask_ranges":u8, "Heading":dbl, "lon":sgl, "lat":sgl, "time":string, "hgps":dbl, "lag":dbl, "MAP":string}
  T2 = cluster{"Steer_input":dbl, "Steer_output":dbl, "handle":dbl}
  T3 = cluster{"VS_des":dbl, "VS_can":dbl, "VS_des":dbl}
  T4 = cluster{"idx":i32, "x":dbl, "y":dbl, "h":dbl, "x_path":dbl}
  T5 = cluster{"idx":i32, "x":dbl, "y":dbl, "hp":dbl, "x_path":dbl}
  T6 = cluster{"X":cluster{"idx":i32, "x":dbl, "y":dbl, "h":dbl, "x_path":dbl}}[]
  T7 = cluster{"GPSTime":dbl, "attitude[2]":dbl, "lcc[0]":dbl, "lcc[1]":dbl, "heading_GPS":dbl}
  T8 = cluster{"Steer_input":dbl, "Steer_output":dbl, "VS_des":dbl, "VS_can":dbl, "heading":dbl, "auto":bool, "run":bool, "x":dbl, "y":dbl}
  T9 = cluster{"Steer_input":dbl, "Steer_output":dbl, dbl}
  T10 = typedef "NI_Matrix.lvlib/RealMatrix.ctl" = dbl[][]
  T11 = cluster{"hash":i64, "sys time":i64, "dt":dbl, "x":dbl, "y":dbl, "speed":dbl, "heading":dbl, "yaw_rate":dbl}
  T12 = cluster{"idx":bool, "x":bool, "y":bool, "h":bool, "x_path":bool}
  T13 = cluster{"idx":dbl, "x":dbl, "y":dbl, "h":dbl, "x_path":dbl}
  T14 = cluster{"c_idx":i32, "xc":dbl, "yc":dbl, "hc":dbl, "xc_path":dbl}
  T15 = cluster{"Minimum":dbl, "Minimum":dbl, "Minimum":dbl, "Minimum":dbl, "Minimum":dbl}
  T16 = cluster{"X":cluster{"c_idx":i32, "xc":dbl, "yc":dbl, "hc":dbl, "xc_path":dbl}}[]
  T17 = cluster{"x":cluster{"idx":i32, "x":dbl, "y":dbl, "h":dbl, "x_path":dbl}}[]
  T18 = cluster{"hash":i64, "sys time":i64, "time":dbl, "x":dbl, "y":dbl, "h":dbl, "numSV":i32, "postype":i32, "lag":i32, "hordev":dbl, "lat":dbl, "lon":dbl, "hgt":dbl, "map_idx":i32}
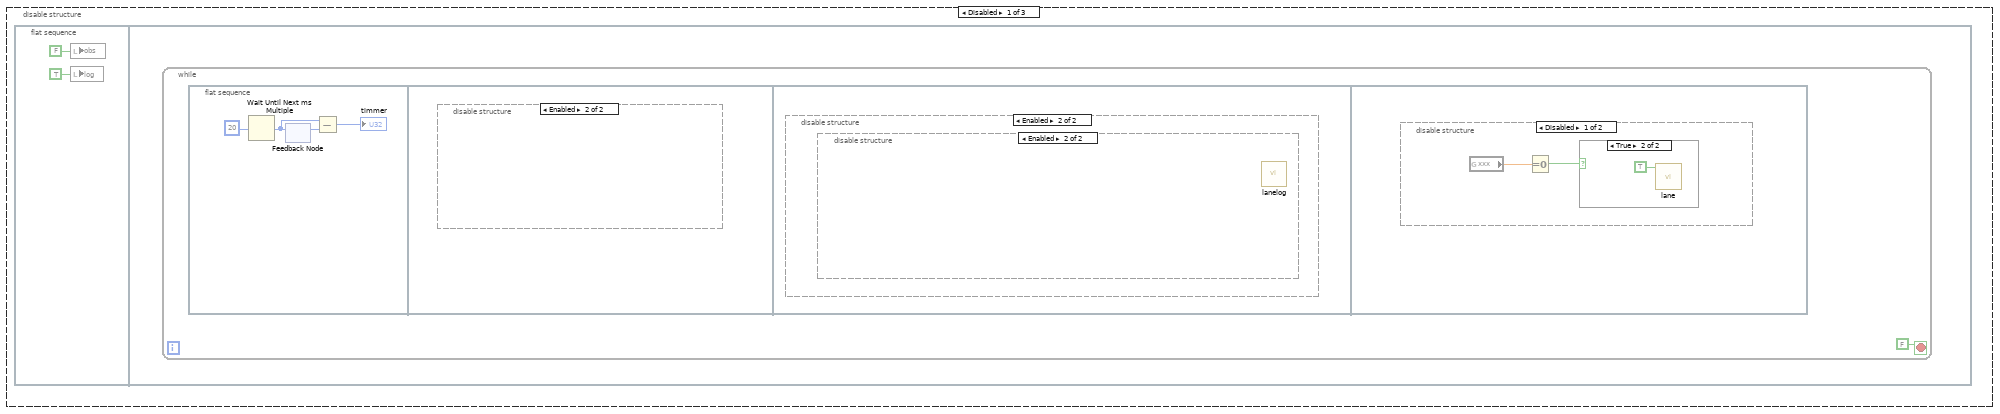
[diagram p2: hidden frame]
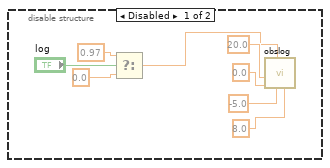
[diagram p3: hidden frame]
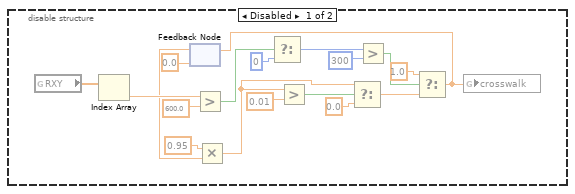
[diagram p5: hidden frame]
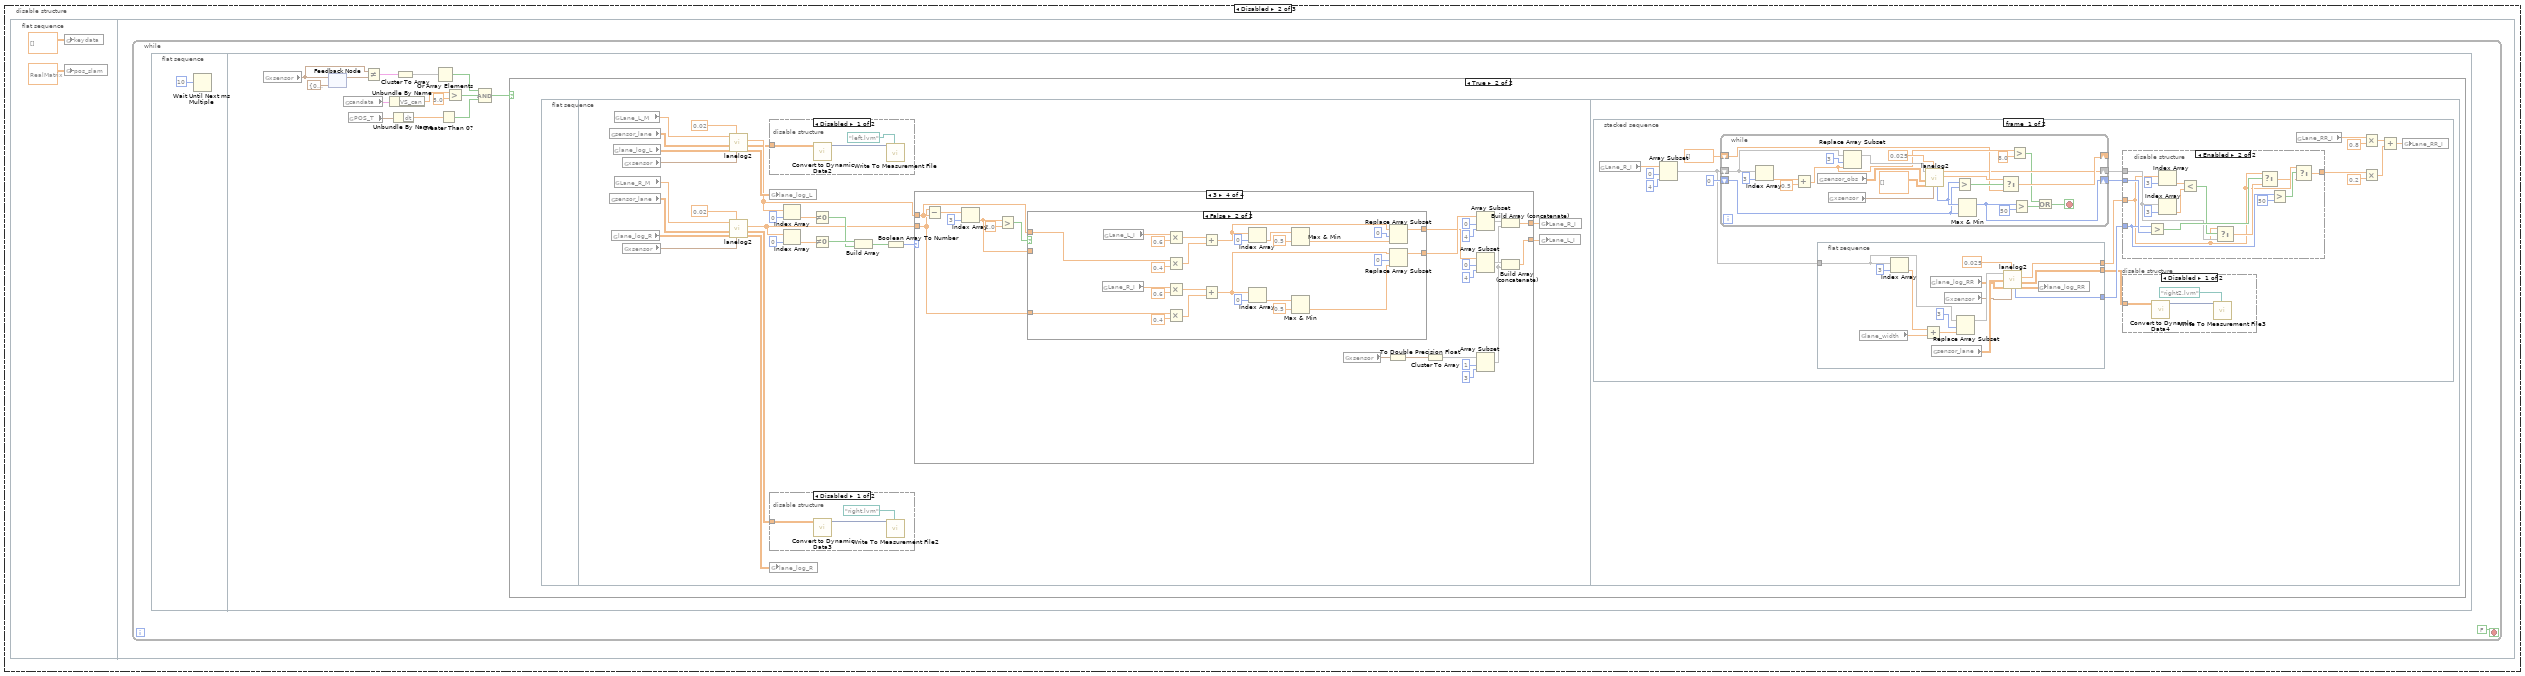
[diagram p8: hidden frame]
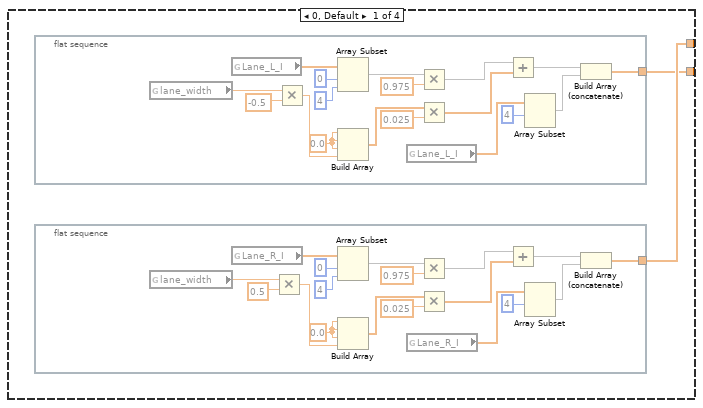
[diagram p12: hidden frame]
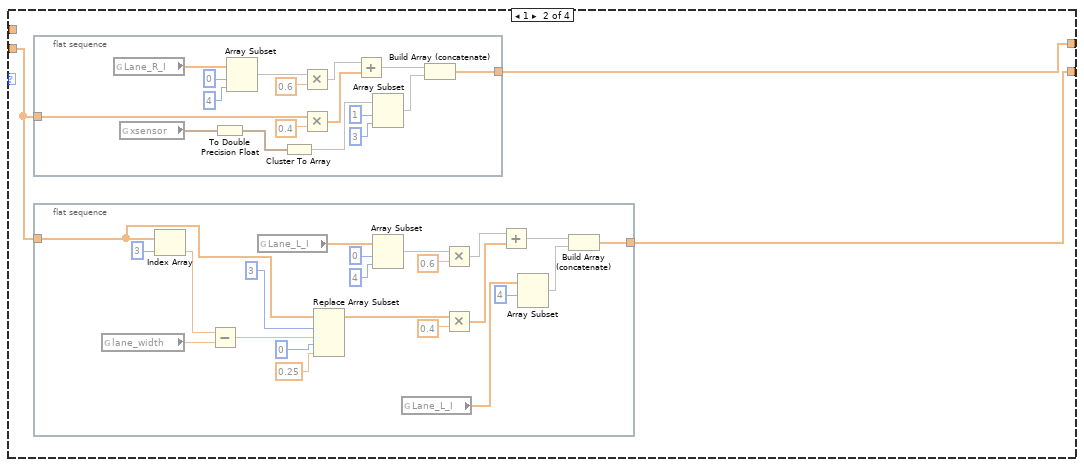
[diagram p13: hidden frame]
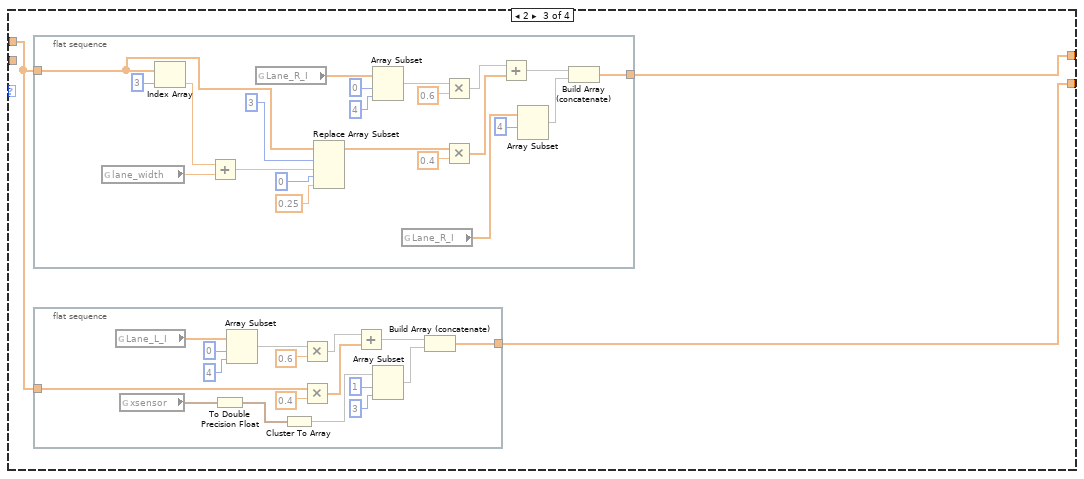
[diagram p14: hidden frame]
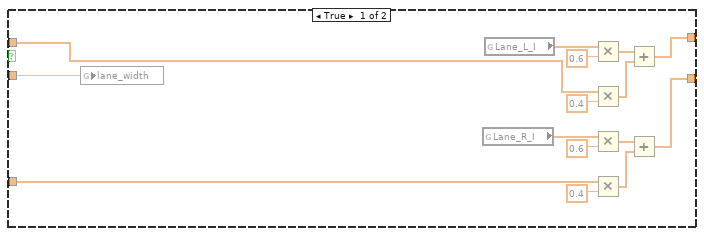
[diagram p15: hidden frame]
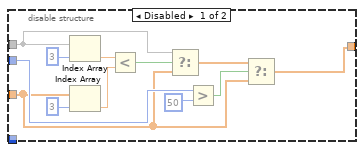
[diagram p17: hidden frame]
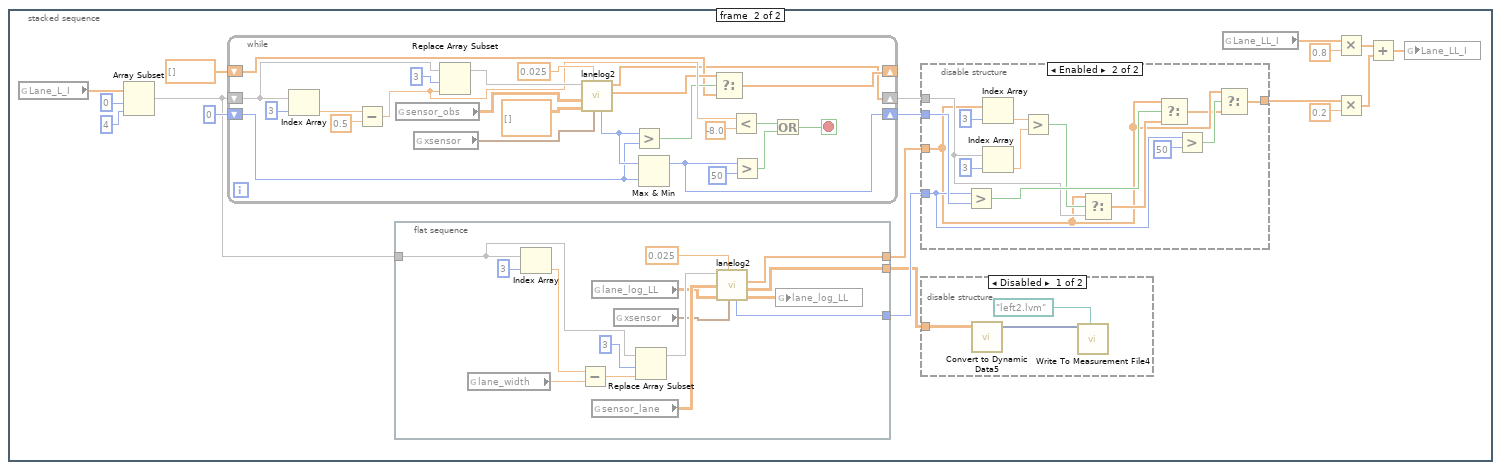
[diagram p18: hidden frame]
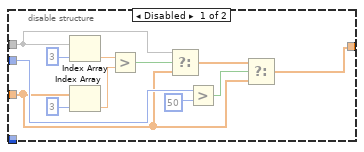
[diagram p20: hidden frame]
diagram:
  n1 = disable-structure shown="Enabled" {
    frame Disabled {
      n2 = call "comm.vi"() -> ()  [unwired: 12 in]
    }
    frame Enabled {
      n3 = call "LCM_data_assign.vi"("time-to-live"=u16 2, "port"=u16 7667) -> ()  [unwired: 10 in]
    }
  }
  n4 = flat-sequence {
    frame #0 {
      # "Control"
    }
    frame #1 {
      w3 = dbl[][] [] ("sensor_car")
      n5 = local write "Reverse"(FALSE ("STOP Signal")) -> ()
      n6 = global write "G_SEN.vi" "data"(w3) -> ()
      n7 = call "initvar.vi"() -> ()  [unwired: 12 in]
      n8 = global write "G_SEN.vi" "sensor_etc"(w3) -> ()
      n9 = global write "G_SEN.vi" "sensor_obs"(w3) -> ()
      n10 = global write "G_SEN.vi" "sensor_lane"(w3) -> ()
    }
    frame #2 {
      n11 = while {
        stop <- FALSE ("Boolean") stop-if-true
        n12 = flat-sequence {
          frame #0 {
            n13 = Wait Until Next ms Multiple(millisecond multiple=u32 10 ("milliseconds to wait")) -> ()  [unwired: 1 out]
          }
          frame #1 {
            n14 = disable-structure shown="Enabled" {
              frame Disabled {
                n15 = global read "G_DATA.vi" "Load data"() -> (w7:bool)
                n16 = case shown="False" w7 {
                  frame False {
                    # "soul"
                    n17 = call "soulpaser.vi"("rionav?"=FALSE) -> ()  [unwired: 11 in]
                  }
                  frame True {
                  }
                }
              }
              frame Disabled {
                n18 = global read "G_DATA.vi" "Load data"() -> (w9:bool)
                n19 = case shown="False" w9 {
                  frame False {
                    # "veloster"
                    n20 = call "velosterpaser.vi"("x"=0.0) -> ()  [unwired: 11 in]
                  }
                  frame True {
                  }
                }
              }
              frame Disabled {
                n21 = global read "G_DATA.vi" "Load data"() -> (w11:bool)
                n22 = case shown="True" w11 {
                  frame False {
                    # "webot"
                    n23 = call "webot.vi"() -> ()  [unwired: 12 in]
                  }
                  frame True {
                  }
                }
              }
              frame Enabled {
                # "LCM"
                n24 = global read "G_LCM.vi" "LCM enable"() -> (w12:bool)
                n25 = case shown="True" w12 {
                  frame False {
                  }
                  frame True {
                    n26 = call "velosterlcmpaser.vi"() -> ()  [unwired: 12 in]
                  }
                }
              }
              frame Disabled {
              }
              frame Disabled {
                # "RCcar"
                n27 = global read "G_DATA.vi" "Load data"() -> (w13:bool)
                n28 = case shown="True" w13 {
                  frame False {
                  }
                  frame True {
                    n29 = global read "G_VEH.vi" "VS_des"() -> (w14:dbl)
                    n30 = global read "G_VEH.vi" "handle"() -> (w15:dbl)
                    n31 = shared-variable "NI-sbRIO9606-01866155\\sharedvari.lvlib\\vs_des"(w14) -> ()  [unwired: 1 in, 1 out]
                    n32 = shared-variable "NI-sbRIO9606-01866155\\sharedvari.lvlib\\steer_input"(w15) -> ()  [unwired: 1 in, 1 out]
                  }
                }
              }
            }
          }
          frame #2 {
            n33 = case shown="False" "RESET PATH" {
              frame False {
                n34 = global read "G_PATH.vi" "path"() -> (w20:dbl[][])
                n35 = global read "G_VEH.vi" "xyhc"() -> (w17:T4)
                n36 = call "findcurrentpointinpath.vi"("xyhc_in"=w17, "path_updated"=w20) -> ("xyhc_out"=w19:T4, "xyhp"=w18:T5)  [unwired: 8 in]
                n37 = global write "G_VEH.vi" "xyhp"(w18) -> ()
                n38 = global write "G_VEH.vi" "xyhc"(w19) -> ()
              }
              frame True {
                n39 = flat-sequence {
                  tunnel: [w26] -> w21
                  tunnel: w21 -> [w33]
                  frame #0 {
                    n40 = call "initvar.vi"() -> ()  [unwired: 12 in]
                  }
                  frame #1 {
                    n41 = global read "G_PATH.vi" "path_very_origin"() -> (w23:dbl[][])
                    n42 = global read "G_PATH.vi" "Missions_origin"() -> (w22:T6)
                    n43 = global write "G_PATH.vi" "path"(w23) -> ()
                    n44 = global write "G_PATH.vi" "Missions"(w22) -> ()
                    n45 = global write "G_PATH.vi" "path_origin"(w23) -> ()
                  }
                  frame #2 {
                    n46 = call "whereami.vi"() -> ()  [unwired: 12 in]
                  }
                  frame #3 {
                    n47 = local write "RESET PATH"(FALSE ("RESET PATH")) -> ()
                  }
                  frame #4 {
                    n48 = global read "G_PATH.vi" "path"() -> (w25:dbl[][])
                    n49 = global read "G_VEH.vi" "xyhc"() -> (w27:T4)
                    n50 = call "findcurrentpointinpath.vi"("xyhc_in"=w27, "path_updated"=w25) -> ("xyhc_out"=w26:T4, "xyhp"=w28:T5)  [unwired: 8 in]
                    n51 = global write "G_VEH.vi" "xyhp"(w28) -> ()
                    n52 = global write "G_VEH.vi" "xyhc"(w26) -> ()
                  }
                  frame #5 {
                    n53 = global write "G_VEH.vi" "xyhc_shift"(w33) -> ()
                    n54 = global read "G_NAV.vi" "M6006"() -> (w31:T7)
                    n55 = Unbundle By Name(w31) -> ("lcc[1]"=w30:dbl, "lcc[0]"=w29:dbl)
                    n56 = Bundle By Name(cluster=w33, "x"=w30, "y"=w29) -> (w32:T4)
                    n57 = global write "G_VEH.vi" "xyhc_lane"(w32) -> ()
                  }
                }
              }
            }
          }
          frame #3 {
            n58 = disable-structure shown="Enabled" {
              frame Enabled {
                n59 = global read "G_VEH.vi" "xyhc_shift"() -> (w43:T4)
                n60 = Unbundle By Name(w43) -> ("x"=w46:dbl, "y"=w48:dbl, "h"=w52:dbl, "idx"=w40:i32)
                n61 = feedback #1(w40) -> (w41:i32)
                n62 = feedback-in #1(w40) -> ()
                n63 = call "headingoperater.vi"("h1"=w52, "h2"=1.5707963267948966) -> ("h2-h1"=w59:dbl)  [unwired: 8 in, 1 out]
                n64 = Equal?(x=w40, y=w41) -> (x = y?=w39:bool)
                n65 = disable-structure shown="Enabled" {
                  disable-tunnel: [w81 _] -> w47
                  disable-tunnel: [w80 _] -> w49
                  frame Enabled {
                    n66 = global read "G_PATH.vi" "xt"() -> (w81:dbl)
                    n67 = global read "G_PATH.vi" "yt"() -> (w80:dbl)
                  }
                  frame Disabled {
                  }
                }
                n68 = case shown="True" w39 {
                  tunnel: [w62 w64] -> w35
                  frame False {
                    w62 = 0.0 ("x")
                    n69 = local write "x"(w62) -> ()
                  }
                  frame True {
                    n70 = local read "x"() -> (w63:dbl)
                    n71 = Multiply(x=w63, y=0.5) -> (x*y=w64:dbl)
                  }
                }
                n72 = global read "G_VEH.vi" "xyhc_lane"() -> (w61:T4)
                n73 = Add(x=w47, y=w46) -> (x+y=w54:dbl)
                n74 = Add(x=w49, y=w48) -> (x+y=w55:dbl)
                n75 = Negate(x=w59) -> (-x=w60:dbl)
                n76 = Unbundle By Name(w61) -> ("x"=w45:dbl, "y"=w44:dbl)
                n77 = global write "G_PATH.vi" "xxx"(w35) -> ()
                n78 = call "rotm_siso.vi"("angle[rad]"=w60, "y0"=w55, "x0"=w54, "y"=w44, "x"=w45) -> ("x'"=w36:dbl)  [unwired: 5 in, 1 out]
                n79 = local read "y"() -> (w34:dbl)
                n80 = Add(x=w36, y=w35) -> (x+y=w42:dbl)
                n81 = Multiply(x=w34, y=0.5) -> (x*y=w37:dbl)
                n82 = call "rotm_siso.vi"("angle[rad]"=w60, "reverse"=TRUE, "y0"=w55, "x0"=w54, "y"=w37, "x"=w42) -> ("y'"=w58:dbl, "x'"=w57:dbl)  [unwired: 4 in]
                n83 = Subtract(x=w57, y=w54) -> (x-y=w50:dbl)
                n84 = Subtract(x=w58, y=w55) -> (x-y=w51:dbl)
                n85 = disable-structure shown="Enabled" {
                  disable-tunnel: w50 -> [w73 _]
                  disable-tunnel: w51 -> [w67 _]
                  frame Enabled {
                    n86 = global read "G_PATH.vi" "yt"() -> (w70:dbl)
                    n87 = global read "G_PATH.vi" "xt"() -> (w77:dbl)
                    n88 = Multiply(x=1.0, y=w70) -> (x*y=w69:dbl)
                    n89 = Multiply(x=1.0, y=w77) -> (x*y=w75:dbl)
                    n90 = Multiply(x=w73, y=0.05 ("x")) -> (x*y=w72:dbl)
                    n91 = Multiply(x=w67, y=0.05 ("x")) -> (x*y=w66:dbl)
                    n92 = Add(x=w75, y=w72) -> (x+y=w79:dbl)
                    n93 = Add(x=w69, y=w66) -> (x+y=w78:dbl)
                    n94 = global write "G_PATH.vi" "xt"(w79) -> ()
                    n95 = global write "G_PATH.vi" "yt"(w78) -> ()
                  }
                  frame Disabled {
                  }
                }
              }
              frame Disabled {
              }
            }
          }
          frame #4 {
            n96 = global read "G_PATH.vi" "Mission"() -> (w82:i32)
            n97 = case shown="0, Default" w82 {
              tunnel: [_ w89] -> w86
              frame 0, Default {
                n98 = global write "G_VEH.vi" "Reverse"(FALSE ("Reverse")) -> ()
              }
              frame 9 {
                n99 = global read "G_VEH.vi" "Reverse"() -> (w89:bool)
              }
            }
            n100 = Select(t="Reverse", s="Reverse", f=w86) -> (s? t:f=w85:bool)
            n101 = call "controller8.vi"("Neg max speed"=-2.0, "reverse"=w85, "slowmode"=FALSE ("slow mode")) -> ()  [unwired: 9 in]
          }
        }
      }
    }
  }
  n102 = flat-sequence {
    frame #0 {
      w90 = FALSE ("LCM")
      # "Display"
      n103 = local write "LCM"(w90) -> ()
      n104 = local write "STOP"(w90) -> ()
    }
    frame #1 {
      n105 = while {
        stop <- FALSE ("exit") stop-if-true
        n106 = flat-sequence {
          frame #0 {
            n107 = Wait Until Next ms Multiple(millisecond multiple=u32 33 ("milliseconds to wait")) -> ()  [unwired: 1 out]
          }
          frame #1 {
            n108 = global read "G_LCM.vi" "recv data"() -> (→"LCM Recv Data":string)
            n109 = Select(t="STOP", s="STOP", f="STOP") -> (s? t:f=w97:bool)
            n110 = Not(x="LCM") -> (.not. x?=w94:bool)
            n111 = global write "G_VEH.vi" "E-STOP"(w97) -> ()
            n112 = global write "G_LCM.vi" "LCM enable"(w94) -> ()
          }
          frame #2 {
            n113 = call "graph2.vi"() -> ("XY Graph"=→"XY Graph":cluster{"Y":dbl[], "Y":dbl[]}[])  [unwired: 10 in, 1 out]
            n114 = call "gpsdata.vi"() -> ("GPS DATA 2"=w100:T1)  [unwired: 11 in]
            "GPS DATA 2" <- w100
            n115 = Unbundle By Name(w100) -> ("Heading"=w102:dbl, "hgps"=w101:dbl)
            n116 = Bundle("Heading"=w102, "hgps"=w101) -> (→"Heading":cluster{"Heading":dbl, "hgps":dbl})  [unwired: 1 in]
          }
          frame #3 {
            n117 = global read "G_VEH.vi" "VS_des"() -> (w104:dbl)
            n118 = Equal To 0?(x=w104) -> (x = 0?=→"stop":bool)
          }
          frame #4 {
            n119 = global read "G_VEH.vi" "candata"() -> (w122:T8)
            n120 = global read "G_VEH.vi" "handle"() -> (w107:dbl)
            n121 = Unbundle By Name(w122) -> ("VS_des"=w114:dbl, "VS_can"=w115:dbl, "run"=w110:bool, "auto"=w111:bool, "Steer_input"=w109:dbl, "Steer_output"=w108:dbl)
            n122 = global read "G_VEH.vi" "VS_des"() -> (w113:dbl)
            n123 = Add(x=w107, y=0.0) -> (x+y=w106:dbl)
            n124 = Not(x=w110) -> (.not. x?=w117:bool)
            n125 = Bundle("VS_des"=w114, "VS_can"=w115, "VS_des"=w113) -> (→"Waveform Chart 2":T3)  [unwired: 1 in]
            n126 = Bundle("VS_des"=w114, "VS_can"=w115, "VS_des"=w113) -> (→"Gauge":T3)  [unwired: 1 in]
            n127 = Bundle("Steer_input"=w109, "Steer_output"=w108, w106) -> (w121:T9)  [unwired: 1 in]
            n128 = Bundle(w117, "auto"=w111) -> (w119:cluster{bool, "auto":bool})  [unwired: 1 in]
            n129 = Negate(x=w121) -> (-x=→"Meter" →"Waveform Chart 3":T9)
            n130 = Boolean To (0,1)(Boolean=w119) -> (0, 1=→"Waveform Chart 4":cluster{i16, "auto":i16})
          }
          frame #5 {
            n131 = global read "G_PATH.vi" "y origin"() -> (w124:dbl[])
            n132 = global read "G_PATH.vi" "x origin"() -> (w125:dbl[])
            n133 = global read "G_NAV.vi" "M6006"() -> (w131:T7)
            n134 = global read "G_VEH.vi" "xyhp"() -> (w123:T4)
            n135 = Unbundle By Name(w131) -> ("lcc[1]"=w132:dbl, "lcc[0]"=w133:dbl)
            n136 = Unbundle By Name(w123) -> ("x"=w127:dbl, "y"=w126:dbl)
            n137 = call "Convert to Dynamic Data6"("Array"=w125) -> ("Dynamic Data Type"=w135:dynamicdata)  [unwired: 3 in]
            n138 = call "Convert to Dynamic Data7"("Array"=w124) -> ("Dynamic Data Type"=w134:dynamicdata)  [unwired: 3 in]
            n139 = Merge Signals(w132, w135, w135, w127) -> (w129:dynamicdata)
            n140 = Merge Signals(w133, w134, w134, w126) -> (w130:dynamicdata)
            n141 = call "GRAPH"("Y Input"=w130, "X Input"=w129) -> ("XY Graph"=→"XY Graph 2":cluster{"Y":dbl[], "Y":dbl[]}[])  [unwired: 3 in, 6 out]
          }
        }
      }
    }
  }
  n142 = disable-structure shown="Enabled" {
    frame Disabled {
      n143 = flat-sequence {
        frame #0 {
          n144 = local write "obs"(FALSE ("obs")) -> ()
          n145 = local write "log"(TRUE ("obs")) -> ()
        }
        frame #1 {
          n146 = while {
            stop <- FALSE stop-if-true
            n147 = flat-sequence {
              frame #0 {
                n148 = Wait Until Next ms Multiple(millisecond multiple=u32 20 ("milliseconds to wait")) -> (millisecond timer value=w142:u32)
                n149 = feedback #2() -> (w140:u32)  [unwired: 1 in]
                n150 = feedback-in #2(w142) -> ()
                n151 = Subtract(x=w142, y=w140) -> (x-y=→"timmer":u32)
              }
              frame #1 {
                n152 = disable-structure shown="Enabled" {
                  frame Disabled {
                    n153 = Select(t=0.97, s="log", f=0.0) -> (s? t:f=w144:dbl)
                    n154 = call "obslog.vi"("xmax"=8.0, "xmin"=-5.0, "FF"=w144, "ymin"=0.0, "ymax"=20.0) -> ()  [unwired: 7 in]
                  }
                  frame Enabled {
                  }
                }
              }
              frame #2 {
                n155 = disable-structure shown="Enabled" {
                  frame Disabled {
                  }
                  frame Enabled {
                    n156 = disable-structure shown="Enabled" {
                      frame Disabled {
                        n157 = global read "G_PATH.vi" "RXY"() -> (w168:dbl[])
                        n158 = Index Array(array=w168) -> (element=w167:dbl)  [unwired: 1 in]
                        n159 = feedback #3(0.0 ("t")) -> (w159:dbl)
                        n160 = Greater?(x=w167, y=600.0) -> (0:w151:bool)
                        n161 = Multiply(x=0.95, y=w159) -> (x*y=w155:dbl)
                        n162 = Select(s=w151, f=i16 0) -> (s? t:f=w163:i16)  [unwired: 1 in]
                        n163 = Greater?(x=w155, y=0.01) -> (0:w156:bool)
                        n164 = Select(t=w155, s=w156, f=0.0) -> (s? t:f=w153:dbl)
                        n165 = Greater?(x=w163, y=i16 300) -> (0:w162:bool)
                        n166 = Select(t=1.0, s=w162, f=w153) -> (s? t:f=w152:dbl)
                        n167 = feedback-in #3(w152) -> ()
                        n168 = global write "G_SEN.vi" "crosswalk"(w152) -> ()
                      }
                      frame Enabled {
                        n169 = call "lanelog.vi"() -> ()  [unwired: 12 in]
                      }
                    }
                  }
                }
              }
              frame #3 {
                n170 = disable-structure shown="Disabled" {
                  frame Disabled {
                    n171 = global read "G_PATH.vi" "xxx"() -> (w170:dbl)
                    n172 = Equal To 0?(x=w170) -> (x = 0?=w169:bool)
                    n173 = case shown="True" w169 {
                      frame False {
                      }
                      frame True {
                        n174 = call "lane.vi"("predict"=TRUE) -> ()  [unwired: 11 in]
                      }
                    }
                  }
                  frame Enabled {
                  }
                }
              }
            }
          }
        }
      }
    }
    frame Disabled {
      n175 = flat-sequence {
        frame #0 {
          n176 = global write "G_SEN.vi" "keydata"(dbl[][] [] ("keydata")) -> ()
          n177 = global write "G_VEH.vi" "pos_slam"(T10 [[1.0, 0.0, 0.0, 0.0], [0.0, 1.0, 0.0, 0.0], [0.0, 0.0, 1.0, 0.0], [0.0, 0.0, 0.0, 1.0]] ("pos_slam")) -> ()
        }
        frame #1 {
          n178 = while {
            stop <- FALSE stop-if-true
            n179 = flat-sequence {
              frame #0 {
                n180 = Wait Until Next ms Multiple(millisecond multiple=u32 10) -> ()  [unwired: 1 out]
              }
              frame #1 {
                n181 = global read "G_VEH.vi" "xsensor"() -> (w187:T4)
                n182 = feedback-in #4(w187) -> ()
                n183 = feedback #4(T4 {"idx"=0, "x"=0.0, "y"=0.0, "h"=0.0, "x_path"=0.0} ("xsensor")) -> (w188:T4)
                n184 = global read "G_VEH.vi" "candata"() -> (w184:T8)
                n185 = global read "G_LCM.vi" "POS_T"() -> (w178:T11)
                n186 = Not Equal?(x=w187, y=w188) -> (x != y?=w186:T12)
                n187 = Unbundle By Name(w184) -> ("VS_can"=w183:dbl)
                n188 = Unbundle By Name(w178) -> ("dt"=w177:dbl)
                n189 = Cluster To Array(cluster=w186) -> (array=w185:bool[])
                n190 = Or Array Elements(Boolean array=w185) -> (logical OR=w181:bool)
                n191 = Greater Than 0?(x=w177) -> (x > 0?=w176:bool)
                n192 = Greater?(x=w183, y=5.0) -> (0:w180:bool)
                n193 = Compound Arithmetic op=AND(w181, w180, w176) -> (w179:bool)
                n194 = case shown="True" w179 {
                  frame False {
                  }
                  frame True {
                    n195 = flat-sequence {
                      frame #0 {
                      }
                      frame #1 {
                        n196 = global read "G_SEN.vi" "sensor_lane"() -> (w200:dbl[][])
                        n197 = global read "G_SEN.vi" "sensor_lane"() -> (w201:dbl[][])
                        n198 = global read "G_SEN.vi" "lane_log_R"() -> (w215:dbl[][])
                        n199 = global read "G_SEN.vi" "lane_log_L"() -> (w212:dbl[][])
                        n200 = global read "G_SEN.vi" "Lane_L_M"() -> (w194:dbl[])
                        n201 = global read "G_SEN.vi" "Lane_R_M"() -> (w195:dbl[])
                        n202 = global read "G_VEH.vi" "xsensor"() -> (w197:T4)
                        n203 = global read "G_VEH.vi" "xsensor"() -> (w196:T4)
                        n204 = call "lanelog2.vi"("xsensor"=w197, "thresh"=0.02, "lane_log"=w212, "sensor"=w200, "Lane_M"=w194) -> ("lane_log_out"=w213:dbl[][], "sensor_out"=w191:dbl[][], "lane_I_out"=w198:dbl[])  [unwired: 2 in, 2 out]
                        n205 = call "lanelog2.vi"("xsensor"=w196, "thresh"=0.02, "lane_log"=w215, "sensor"=w201, "Lane_M"=w195) -> ("lane_log_out"=w214:dbl[][], "sensor_out"=w190:dbl[][], "lane_I_out"=w199:dbl[])  [unwired: 2 in, 2 out]
                        n206 = disable-structure shown="Disabled" {
                          disable-tunnel: w191 -> [w217 _]
                          frame Disabled {
                            n207 = call "Convert to Dynamic Data2"("2D Array"=w217) -> ("Dynamic Data Type"=w218:dynamicdata)  [unwired: 3 in]
                            n208 = call "Write To Measurement File"("Signals"=w218, "Filename"=path "left.lvm") -> ()  [unwired: 15 in, 3 out]
                          }
                          frame Enabled {
                          }
                        }
                        n209 = global write "G_SEN.vi" "lane_log_L"(w213) -> ()
                        n210 = disable-structure shown="Disabled" {
                          disable-tunnel: w190 -> [w219 _]
                          frame Disabled {
                            n211 = call "Convert to Dynamic Data3"("2D Array"=w219) -> ("Dynamic Data Type"=w220:dynamicdata)  [unwired: 3 in]
                            n212 = call "Write To Measurement File2"("Signals"=w220, "Filename"=path "right.lvm") -> ()  [unwired: 15 in, 3 out]
                          }
                          frame Enabled {
                          }
                        }
                        n213 = global write "G_SEN.vi" "lane_log_R"(w214) -> ()
                        n214 = Index Array(array=w198, index=0) -> (element=w209:dbl)
                        n215 = Index Array(array=w199, index=0) -> (element=w210:dbl)
                        n216 = Not Equal To 0?(x=w209) -> (x != 0?=w206:bool)
                        n217 = Not Equal To 0?(x=w210) -> (x != 0?=w207:bool)
                        n218 = Build Array(w207, w206) -> (w205:bool[])
                        n219 = Boolean Array To Number(Boolean array=w205) -> (number=w204:u32)
                        n220 = case shown="3" w204 {
                          tunnel: w199 -> [_ w262 _ w363]
                          tunnel: w198 -> [_ _ w304 w364]
                          tunnel: [w223 w261 w302 w355] -> w193
                          tunnel: [w222 w260 w303 w345] -> w192
                          frame 0, Default {
                            n221 = flat-sequence {
                              tunnel: [w224] -> w222
                              frame #0 {
                                w237 = 0.0 ("element")
                                n222 = global read "G_SEN.vi" "lane_width"() -> (w236:dbl)
                                n223 = global read "G_SEN.vi" "Lane_L_I"() -> (w230:dbl[])
                                n224 = Multiply(x=w236, y=-0.5) -> (x*y=w234:dbl)
                                n225 = Array Subset(array=w230, index=0, length=4) -> (w229:dbl[])
                                n226 = Build Array(w237, w237, w237, w234) -> (w233:dbl[])
                                n227 = global read "G_SEN.vi" "Lane_L_I"() -> (w228:dbl[])
                                n228 = Multiply(x=w229, y=0.975) -> (x*y=w239:dbl[])
                                n229 = Multiply(x=w233, y=0.025) -> (x*y=w238:dbl[])
                                n230 = Add(x=w239, y=w238) -> (x+y=w226:dbl[])
                                n231 = Array Subset(array=w228, index=4) -> (w225:dbl[])  [unwired: 1 in]
                                n232 = Build Array (concatenate)(w226, w225) -> (w224:dbl[])
                              }
                            }
                            n233 = flat-sequence {
                              tunnel: [w242] -> w223
                              frame #0 {
                                w255 = 0.0 ("element")
                                n234 = global read "G_SEN.vi" "lane_width"() -> (w256:dbl)
                                n235 = global read "G_SEN.vi" "Lane_R_I"() -> (w248:dbl[])
                                n236 = Multiply(x=w256, y=0.5) -> (x*y=w258:dbl)
                                n237 = Array Subset(array=w248, index=0, length=4) -> (w247:dbl[])
                                n238 = Build Array(w255, w255, w255, w258) -> (w259:dbl[])
                                n239 = global read "G_SEN.vi" "Lane_R_I"() -> (w246:dbl[])
                                n240 = Multiply(x=w247, y=0.975) -> (x*y=w253:dbl[])
                                n241 = Multiply(x=w259, y=0.025) -> (x*y=w254:dbl[])
                                n242 = Add(x=w253, y=w254) -> (x+y=w244:dbl[])
                                n243 = Array Subset(array=w246, index=4) -> (w243:dbl[])  [unwired: 1 in]
                                n244 = Build Array (concatenate)(w244, w243) -> (w242:dbl[])
                              }
                            }
                          }
                          frame 1 {
                            n245 = flat-sequence {
                              tunnel: w262 -> [w297]
                              tunnel: [w285] -> w261
                              frame #0 {
                                n246 = global read "G_SEN.vi" "Lane_R_I"() -> (w294:dbl[])
                                n247 = global read "G_VEH.vi" "xsensor"() -> (w292:T4)
                                n248 = To Double Precision Float(number=w292) -> (double precision float=w291:T13)
                                n249 = Array Subset(array=w294, index=0, length=4) -> (w293:dbl[])
                                n250 = Cluster To Array(cluster=w291) -> (array=w290:dbl[])
                                n251 = Multiply(x=w293, y=0.6) -> (x*y=w299:dbl[])
                                n252 = Multiply(x=w297, y=0.4) -> (x*y=w298:dbl[])
                                n253 = Add(x=w299, y=w298) -> (x+y=w286:dbl[])
                                n254 = Array Subset(array=w290, index=1, length=3) -> (w287:dbl[])
                                n255 = Build Array (concatenate)(w286, w287) -> (w285:dbl[])
                              }
                            }
                            n256 = flat-sequence {
                              tunnel: w262 -> [w277]
                              tunnel: [w263] -> w260
                              frame #0 {
                                n257 = global read "G_SEN.vi" "lane_width"() -> (w282:dbl)
                                n258 = Index Array(array=w277, index=3) -> (element=w283:dbl)
                                n259 = Subtract(x=w283, y=w282) -> (x-y=w280:dbl)
                                n260 = global read "G_SEN.vi" "Lane_L_I"() -> (w267:dbl[])
                                n261 = Replace Array Subset(array=w277, new element #1=w280, index #1=3 ("index"), new element #2=0.25 ("new element/subarray"), index #2=0 ("index")) -> (w272:dbl[])
                                n262 = Array Subset(array=w267, index=0, length=4) -> (w269:dbl[])
                                n263 = global read "G_SEN.vi" "Lane_L_I"() -> (w264:dbl[])
                                n264 = Multiply(x=w269, y=0.6) -> (x*y=w275:dbl[])
                                n265 = Multiply(x=w272, y=0.4) -> (x*y=w276:dbl[])
                                n266 = Add(x=w275, y=w276) -> (x+y=w266:dbl[])
                                n267 = Array Subset(array=w264, index=4) -> (w265:dbl[])  [unwired: 1 in]
                                n268 = Build Array (concatenate)(w266, w265) -> (w263:dbl[])
                              }
                            }
                          }
                          frame 2 {
                            n269 = flat-sequence {
                              tunnel: w304 -> [w319]
                              tunnel: [w305] -> w302
                              frame #0 {
                                n270 = global read "G_SEN.vi" "lane_width"() -> (w324:dbl)
                                n271 = Index Array(array=w319, index=3) -> (element=w325:dbl)
                                n272 = Add(x=w325, y=w324) -> (x+y=w322:dbl)
                                n273 = global read "G_SEN.vi" "Lane_R_I"() -> (w312:dbl[])
                                n274 = Replace Array Subset(array=w319, new element #1=w322, index #1=3 ("index"), new element #2=0.25 ("new element/subarray"), index #2=0 ("index")) -> (w314:dbl[])
                                n275 = Array Subset(array=w312, index=0, length=4) -> (w310:dbl[])
                                n276 = global read "G_SEN.vi" "Lane_R_I"() -> (w309:dbl[])
                                n277 = Multiply(x=w310, y=0.6) -> (x*y=w316:dbl[])
                                n278 = Multiply(x=w314, y=0.4) -> (x*y=w315:dbl[])
                                n279 = Add(x=w316, y=w315) -> (x+y=w306:dbl[])
                                n280 = Array Subset(array=w309, index=4) -> (w307:dbl[])  [unwired: 1 in]
                                n281 = Build Array (concatenate)(w306, w307) -> (w305:dbl[])
                              }
                            }
                            n282 = flat-sequence {
                              tunnel: w304 -> [w339]
                              tunnel: [w327] -> w303
                              frame #0 {
                                n283 = global read "G_SEN.vi" "Lane_L_I"() -> (w336:dbl[])
                                n284 = global read "G_VEH.vi" "xsensor"() -> (w334:T4)
                                n285 = To Double Precision Float(number=w334) -> (double precision float=w333:T13)
                                n286 = Array Subset(array=w336, index=0, length=4) -> (w335:dbl[])
                                n287 = Cluster To Array(cluster=w333) -> (array=w332:dbl[])
                                n288 = Multiply(x=w335, y=0.6) -> (x*y=w341:dbl[])
                                n289 = Multiply(x=w339, y=0.4) -> (x*y=w340:dbl[])
                                n290 = Add(x=w341, y=w340) -> (x+y=w329:dbl[])
                                n291 = Array Subset(array=w332, index=1, length=3) -> (w328:dbl[])
                                n292 = Build Array (concatenate)(w329, w328) -> (w327:dbl[])
                              }
                            }
                          }
                          frame 3 {
                            n293 = Subtract(x=w363, y=w364) -> (x-y=w366:dbl[])
                            n294 = Index Array(array=w366, index=3) -> (element=w361:dbl)
                            n295 = Greater?(x=w361, y=2.0) -> (0:w360:bool)
                            n296 = case shown="False" w360 {
                              tunnel: w364 -> [w376 w402]
                              tunnel: [w375 w394] -> w346
                              tunnel: w363 -> [w369 w396]
                              tunnel: [w368 w392] -> w356
                              tunnel: w361 -> [w367 _]
                              frame True {
                                n297 = global write "G_SEN.vi" "lane_width"(w367) -> ()
                                n298 = global read "G_SEN.vi" "Lane_R_I"() -> (w370:dbl[])
                                n299 = global read "G_SEN.vi" "Lane_L_I"() -> (w377:dbl[])
                                n300 = Multiply(x=w377, y=0.6) -> (x*y=w379:dbl[])
                                n301 = Multiply(x=w376, y=0.4) -> (x*y=w378:dbl[])
                                n302 = Multiply(x=w370, y=0.6) -> (x*y=w372:dbl[])
                                n303 = Multiply(x=w369, y=0.4) -> (x*y=w371:dbl[])
                                n304 = Add(x=w379, y=w378) -> (x+y=w375:dbl[])
                                n305 = Add(x=w372, y=w371) -> (x+y=w368:dbl[])
                              }
                              frame False {
                                n306 = global read "G_SEN.vi" "Lane_R_I"() -> (w397:dbl[])
                                n307 = global read "G_SEN.vi" "Lane_L_I"() -> (w403:dbl[])
                                n308 = Multiply(x=w403, y=0.6) -> (x*y=w405:dbl[])
                                n309 = Multiply(x=w402, y=0.4) -> (x*y=w404:dbl[])
                                n310 = Multiply(x=w397, y=0.6) -> (x*y=w399:dbl[])
                                n311 = Multiply(x=w396, y=0.4) -> (x*y=w398:dbl[])
                                n312 = Add(x=w405, y=w404) -> (x+y=w382:dbl[])
                                n313 = Add(x=w399, y=w398) -> (x+y=w391:dbl[])
                                n314 = Index Array(array=w382, index=0) -> (element=w385:dbl)
                                n315 = Index Array(array=w391, index=0) -> (element=w389:dbl)
                                n316 = Max & Min(x=w385, y=0.5 ("new element/subarray")) -> (min(x,y)=w383:dbl)  [unwired: 1 out]
                                n317 = Max & Min(x=w389, y=0.5 ("new element/subarray")) -> (min(x,y)=w387:dbl)  [unwired: 1 out]
                                n318 = Replace Array Subset(array=w382, new element=w383, index=0) -> (w394:dbl[])
                                n319 = Replace Array Subset(array=w391, new element=w387, index=0) -> (w392:dbl[])
                              }
                            }
                            n320 = global read "G_VEH.vi" "xsensor"() -> (w354:T4)
                            n321 = To Double Precision Float(number=w354) -> (double precision float=w353:T13)
                            n322 = Cluster To Array(cluster=w353) -> (array=w352:dbl[])
                            n323 = Array Subset(array=w356, index=0, length=4) -> (w357:dbl[])
                            n324 = Array Subset(array=w346, index=0, length=4) -> (w349:dbl[])
                            n325 = Array Subset(array=w352, index=1, length=3) -> (w344:dbl[])
                            n326 = Build Array (concatenate)(w357, w344) -> (w355:dbl[])
                            n327 = Build Array (concatenate)(w349, w344) -> (w345:dbl[])
                          }
                        }
                        n328 = global write "G_SEN.vi" "Lane_R_I"(w193) -> ()
                        n329 = global write "G_SEN.vi" "Lane_L_I"(w192) -> ()
                      }
                      frame #2 {
                        n330 = stacked-sequence {
                          frame #0 {
                            n331 = global read "G_SEN.vi" "Lane_R_I"() -> (w410:dbl[])
                            n332 = Array Subset(array=w410, index=0, length=4) -> (w409:dbl[])
                            n333 = while {
                              shift-right: [w482] -> _
                              shift-left: dbl[] [] ("lane_I_out") -> [w481]
                              shift-right: [w472] -> w423
                              shift-left: 0 ("size") -> [w479]
                              shift-right: [w477] -> w422
                              shift-left: w409 -> [w478]
                              stop <- w473 stop-if-true
                              n334 = Index Array(array=w478, index=3) -> (element=w490:dbl)
                              n335 = Add(x=w490, y=0.5) -> (x+y=w486:dbl)
                              n336 = global read "G_SEN.vi" "sensor_obs"() -> (w494:dbl[][])
                              n337 = global read "G_VEH.vi" "xsensor"() -> (w471:T4)
                              n338 = Replace Array Subset(array=w478, new element=w486, index=3) -> (w492:dbl[])
                              n339 = call "lanelog2.vi"("xsensor"=w471, "thresh"=0.025, "lane_log"=dbl[][] [], "sensor"=w494, "Lane_M"=w492) -> ("lane_I_out"=w483:dbl[], "lane_M_out"=w477:dbl[], "size"=w480:i32)  [unwired: 2 in, 2 out]
                              n340 = Greater?(x=w480, y=w479) -> (0:w484:bool)
                              n341 = Max & Min(x=w480, y=w479) -> (max(x,y)=w472:i32)  [unwired: 1 out]
                              n342 = Select(t=w483, s=w484, f=w481) -> (s? t:f=w482:dbl[])
                              n343 = Greater?(x=w486, y=8.0) -> (0:w474:bool)
                              n344 = Greater?(x=w472, y=50) -> (0:w475:bool)
                              n345 = Or(x=w474, y=w475) -> (x .or. y?=w473:bool)
                            }
                            n346 = flat-sequence {
                              tunnel: [w460] -> w421
                              tunnel: [w459] -> w420
                              tunnel: w409 -> [w457]
                              tunnel: [w456] -> w408
                              frame #0 {
                                n347 = global read "G_SEN.vi" "lane_width"() -> (w465:dbl)
                                n348 = Index Array(array=w457, index=3) -> (element=w466:dbl)
                                n349 = Add(x=w466, y=w465) -> (x+y=w463:dbl)
                                n350 = global read "G_SEN.vi" "lane_log_RR"() -> (w461:dbl[][])
                                n351 = global read "G_SEN.vi" "sensor_lane"() -> (w470:dbl[][])
                                n352 = global read "G_VEH.vi" "xsensor"() -> (w458:T4)
                                n353 = Replace Array Subset(array=w457, new element=w463, index=3) -> (w468:dbl[])
                                n354 = call "lanelog2.vi"("xsensor"=w458, "thresh"=0.025, "lane_log"=w461, "sensor"=w470, "Lane_M"=w468) -> ("lane_log_out"=w462:dbl[][], "sensor_out"=w456:dbl[][], "lane_I_out"=w460:dbl[], "size"=w459:i32)  [unwired: 2 in, 1 out]
                                n355 = global write "G_SEN.vi" "lane_log_RR"(w462) -> ()
                              }
                            }
                            n356 = disable-structure shown="Enabled" {
                              disable-tunnel: w423 -> [w439 w455]
                              disable-tunnel: [w437 w441] -> w414
                              disable-tunnel: w422 -> [w431 w448]
                              disable-tunnel: w421 -> [w430 w443]
                              disable-tunnel: w420 -> [_ w446]
                              frame Disabled {
                                n357 = Index Array(array=w431, index=3) -> (element=w434:dbl)
                                n358 = Index Array(array=w430, index=3) -> (element=w433:dbl)
                                n359 = Less?(x=w434, y=w433) -> (x < y?=w432:bool)
                                n360 = Select(t=w431, s=w432, f=w430) -> (s? t:f=w429:dbl[])
                                n361 = Greater?(x=w439, y=50) -> (0:w438:bool)
                                n362 = Select(t=w429, s=w438, f=w430) -> (s? t:f=w437:dbl[])
                              }
                              frame Enabled {
                                n363 = Greater?(x=w446, y=w455) -> (0:w454:bool)
                                n364 = Index Array(array=w443, index=3) -> (element=w451:dbl)
                                n365 = Index Array(array=w448, index=3) -> (element=w450:dbl)
                                n366 = Less?(x=w451, y=w450) -> (x < y?=w449:bool)
                                n367 = Select(t=w443, s=w449, f=w448) -> (s? t:f=w447:dbl[])
                                n368 = Select(t=w443, s=w454, f=w447) -> (s? t:f=w442:dbl[])
                                n369 = Greater?(x=w446, y=50) -> (0:w444:bool)
                                n370 = Select(t=w443, s=w444, f=w442) -> (s? t:f=w441:dbl[])
                              }
                            }
                            n371 = disable-structure shown="Disabled" {
                              disable-tunnel: w408 -> [w426 _]
                              frame Disabled {
                                n372 = call "Convert to Dynamic Data4"("2D Array"=w426) -> ("Dynamic Data Type"=w428:dynamicdata)  [unwired: 3 in]
                                n373 = call "Write To Measurement File3"("Signals"=w428, "Filename"=path "right2.lvm") -> ()  [unwired: 15 in, 3 out]
                              }
                              frame Enabled {
                              }
                            }
                            n374 = global read "G_SEN.vi" "Lane_RR_I"() -> (w415:dbl[])
                            n375 = Multiply(x=w415, y=0.8) -> (x*y=w417:dbl[])
                            n376 = Multiply(x=w414, y=0.2) -> (x*y=w416:dbl[])
                            n377 = Add(x=w417, y=w416) -> (x+y=w413:dbl[])
                            n378 = global write "G_SEN.vi" "Lane_RR_I"(w413) -> ()
                          }
                          frame #1 {
                            n379 = global read "G_SEN.vi" "Lane_L_I"() -> (w497:dbl[])
                            n380 = Array Subset(array=w497, index=0, length=4) -> (w496:dbl[])
                            n381 = while {
                              shift-right: [w569] -> _
                              shift-left: dbl[] [] ("lane_I_out") -> [w568]
                              shift-right: [w559] -> w510
                              shift-left: 0 ("size") -> [w566]
                              shift-right: [w564] -> w509
                              shift-left: w496 -> [w565]
                              stop <- w560 stop-if-true
                              n382 = Index Array(array=w565, index=3) -> (element=w577:dbl)
                              n383 = Subtract(x=w577, y=0.5) -> (x-y=w573:dbl)
                              n384 = global read "G_SEN.vi" "sensor_obs"() -> (w581:dbl[][])
                              n385 = global read "G_VEH.vi" "xsensor"() -> (w558:T4)
                              n386 = Replace Array Subset(array=w565, new element=w573, index=3) -> (w579:dbl[])
                              n387 = call "lanelog2.vi"("xsensor"=w558, "thresh"=0.025, "lane_log"=dbl[][] [], "sensor"=w581, "Lane_M"=w579) -> ("lane_I_out"=w570:dbl[], "lane_M_out"=w564:dbl[], "size"=w567:i32)  [unwired: 2 in, 2 out]
                              n388 = Greater?(x=w567, y=w566) -> (0:w571:bool)
                              n389 = Max & Min(x=w567, y=w566) -> (max(x,y)=w559:i32)  [unwired: 1 out]
                              n390 = Select(t=w570, s=w571, f=w568) -> (s? t:f=w569:dbl[])
                              n391 = Less?(x=w573, y=-8.0) -> (x < y?=w561:bool)
                              n392 = Greater?(x=w559, y=50) -> (0:w562:bool)
                              n393 = Or(x=w561, y=w562) -> (x .or. y?=w560:bool)
                            }
                            n394 = flat-sequence {
                              tunnel: [w547] -> w508
                              tunnel: [w546] -> w507
                              tunnel: w496 -> [w544]
                              tunnel: [w543] -> w495
                              frame #0 {
                                n395 = global read "G_SEN.vi" "lane_width"() -> (w552:dbl)
                                n396 = Index Array(array=w544, index=3) -> (element=w553:dbl)
                                n397 = Subtract(x=w553, y=w552) -> (x-y=w550:dbl)
                                n398 = global read "G_SEN.vi" "lane_log_LL"() -> (w548:dbl[][])
                                n399 = global read "G_SEN.vi" "sensor_lane"() -> (w557:dbl[][])
                                n400 = global read "G_VEH.vi" "xsensor"() -> (w545:T4)
                                n401 = Replace Array Subset(array=w544, new element=w550, index=3) -> (w555:dbl[])
                                n402 = call "lanelog2.vi"("xsensor"=w545, "thresh"=0.025, "lane_log"=w548, "sensor"=w557, "Lane_M"=w555) -> ("lane_log_out"=w549:dbl[][], "sensor_out"=w543:dbl[][], "lane_I_out"=w547:dbl[], "size"=w546:i32)  [unwired: 2 in, 1 out]
                                n403 = global write "G_SEN.vi" "lane_log_LL"(w549) -> ()
                              }
                            }
                            n404 = disable-structure shown="Enabled" {
                              disable-tunnel: w510 -> [w526 w542]
                              disable-tunnel: [w524 w528] -> w503
                              disable-tunnel: w509 -> [w518 w535]
                              disable-tunnel: w508 -> [w517 w530]
                              disable-tunnel: w507 -> [_ w533]
                              frame Disabled {
                                n405 = Index Array(array=w518, index=3) -> (element=w521:dbl)
                                n406 = Index Array(array=w517, index=3) -> (element=w520:dbl)
                                n407 = Greater?(x=w521, y=w520) -> (0:w519:bool)
                                n408 = Select(t=w518, s=w519, f=w517) -> (s? t:f=w516:dbl[])
                                n409 = Greater?(x=w526, y=50) -> (0:w525:bool)
                                n410 = Select(t=w516, s=w525, f=w517) -> (s? t:f=w524:dbl[])
                              }
                              frame Enabled {
                                n411 = Greater?(x=w533, y=w542) -> (0:w541:bool)
                                n412 = Index Array(array=w530, index=3) -> (element=w538:dbl)
                                n413 = Index Array(array=w535, index=3) -> (element=w537:dbl)
                                n414 = Greater?(x=w538, y=w537) -> (0:w536:bool)
                                n415 = Select(t=w530, s=w536, f=w535) -> (s? t:f=w534:dbl[])
                                n416 = Select(t=w530, s=w541, f=w534) -> (s? t:f=w529:dbl[])
                                n417 = Greater?(x=w533, y=50) -> (0:w531:bool)
                                n418 = Select(t=w530, s=w531, f=w529) -> (s? t:f=w528:dbl[])
                              }
                            }
                            n419 = disable-structure shown="Disabled" {
                              disable-tunnel: w495 -> [w513 _]
                              frame Disabled {
                                n420 = call "Convert to Dynamic Data5"("2D Array"=w513) -> ("Dynamic Data Type"=w514:dynamicdata)  [unwired: 3 in]
                                n421 = call "Write To Measurement File4"("Signals"=w514, "Filename"=path "left2.lvm") -> ()  [unwired: 15 in, 3 out]
                              }
                              frame Enabled {
                              }
                            }
                            n422 = global read "G_SEN.vi" "Lane_LL_I"() -> (w506:dbl[])
                            n423 = Multiply(x=w506, y=0.8) -> (x*y=w502:dbl[])
                            n424 = Multiply(x=w503, y=0.2) -> (x*y=w501:dbl[])
                            n425 = Add(x=w502, y=w501) -> (x+y=w500:dbl[])
                            n426 = global write "G_SEN.vi" "Lane_LL_I"(w500) -> ()
                          }
                        }
                      }
                    }
                  }
                }
              }
            }
          }
        }
      }
    }
    frame Enabled {
      n427 = while {
        stop <- FALSE stop-if-true
        n428 = flat-sequence {
          tunnel: [w585] -> w582
          tunnel: w582 -> [w623]
          frame #0 {
            n429 = Wait Until Next ms Multiple(millisecond multiple=u32 10) -> ()  [unwired: 1 out]
          }
          frame #1 {
            n430 = flat-sequence {
              tunnel: [w596] -> w590
              tunnel: [w595] -> w589
              tunnel: [w594] -> w588
              tunnel: [w593] -> w587
              tunnel: [w591] -> w586
              frame #0 {
                w592 = TRUE ("Sensor [F12]")
                n431 = call "velodynepaser.vi"() -> ()  [unwired: 9 in, 3 out]
                n432 = call "Ibeopaser.vi"("Hide Transparent"=w592, "Sensor [F12]"=w592) -> ("x_sensor"=w595:T4, "etc"=w593:dbl[][], "lane"=w594:dbl[][], "obs"=w596:dbl[][], "update"=w591:bool)  [unwired: 5 in]
                n433 = call "mobileyepaser.vi"() -> ()  [unwired: 11 in, 1 out]
              }
            }
            n434 = case shown="True" w586 {
              tunnel: w590 -> [_ w604]
              tunnel: w589 -> [_ w603]
              tunnel: w588 -> [_ w602]
              tunnel: w587 -> [_ w601]
              tunnel: [w597 w600] -> w585
              frame False {
                n435 = global read "G_SEN.vi" "sensor_lane_log"() -> (w599:dbl[][])
                n436 = global read "G_VEH.vi" "xsensor"() -> (w598:T4)
                n437 = call "sensor_log.vi"("xsensor"=w598, "sensor_log"=w599) -> ("sensor_log_body"=w597:dbl[][])  [unwired: 7 in, 2 out]
              }
              frame True {
                n438 = flat-sequence {
                  tunnel: w604 -> [w608]
                  tunnel: w603 -> [w607]
                  tunnel: w602 -> [w606]
                  tunnel: w601 -> [w605]
                  tunnel: [w617] -> w600
                  frame #0 {
                    n439 = global write "G_SEN.vi" "sensor_obs"(w608) -> ()
                    n440 = global write "G_SEN.vi" "sensor_lane"(w606) -> ()
                    n441 = global write "G_SEN.vi" "sensor_etc"(w605) -> ()
                    n442 = global write "G_VEH.vi" "xsensor"(w607) -> ()
                  }
                  frame #1 {
                    n443 = global read "G_VEH.vi" "candata"() -> (w610:T8)
                    n444 = global read "G_LCM.vi" "POS_T"() -> (w614:T11)
                    n445 = Unbundle By Name(w610) -> ("VS_can"=w611:dbl)
                    n446 = Unbundle By Name(w614) -> ("dt"=w615:dbl)
                    n447 = global read "G_SEN.vi" "sensor_lane_log"() -> (w620:dbl[][])
                    n448 = global read "G_SEN.vi" "sensor_lane"() -> (w621:dbl[][])
                    n449 = global read "G_VEH.vi" "xsensor"() -> (w618:T4)
                    n450 = Greater Than 0?(x=w615) -> (x > 0?=w616:bool)
                    n451 = Greater?(x=w611, y=5.0) -> (0:w613:bool)
                    n452 = call "sensor_log.vi"("xsensor"=w618, "sensor_log"=w620, "sensor"=w621) -> ("sensor_log_out"=w619:dbl[][], "sensor_log_body"=w617:dbl[][])  [unwired: 6 in, 1 out]
                    n453 = Compound Arithmetic op=AND(w613, w616) -> (w609:bool)
                    n454 = case shown="True" w609 {
                      tunnel: w619 -> [_ w622]
                      frame False {
                      }
                      frame True {
                        n455 = global write "G_SEN.vi" "sensor_lane_log"(w622) -> ()
                      }
                    }
                  }
                }
              }
            }
          }
          frame #2 {
            n456 = disable-structure shown="Disabled" {
              disable-tunnel: w623 -> [w624 _]
              frame Disabled {
                n457 = call "obs2lane2.vi"("sensors inputs"=w624) -> ()  [unwired: 11 in]
              }
              frame Enabled {
              }
            }
          }
        }
      }
    }
  }
  n458 = flat-sequence {
    frame #0 {
      # "1. Alogorithm\n2. Make & Laod path"
    }
    frame #1 {
      w637 = FALSE ("Make WPT")
      n459 = global write "G_VEH.vi" "handle"(0.0 ("handle")) -> ()
      n460 = local write "mobileye"(TRUE ("mobileye")) -> ()
      n461 = global write "G_PATH.vi" "lane_init"(FALSE ("lane_init")) -> ()
      n462 = global write "G_VEH.vi" "firstcall"(FALSE ("firstcall")) -> ()
      n463 = Current VI's Path() -> (path=w633:path)
      n464 = global write "G_SEN.vi" "lane_m_R"(1.75 ("lane_m_R")) -> ()
      n465 = global write "G_SEN.vi" "lane_m_L"(-1.75 ("lane_m_L")) -> ()
      n466 = local write "Make WPT"(w637) -> ()
      n467 = local write "Load WPT"(w637) -> ()
      n468 = global write "G_SEN.vi" "sensor_lane_log"(dbl[][] [] ("sensor_lane_log")) -> ()
      n469 = for {
        N: 500 -> [_]
        tunnel: [w638] -> w627 mode=indexing
        i -> [w641]
        n470 = To Double Precision Float(number=w641) -> (double precision float=w640:dbl)
        n471 = Multiply(x=0.1, y=w640) -> (x*y=w638:dbl)
      }
      n472 = Strip Path(path=w633) -> (stripped path=w632:path)  [unwired: 1 out]
      n473 = global write "G_DATA.vi" "path"(w632) -> ()
      n474 = local write "x"(0.0 ("x")) -> ()
      n475 = global write "G_SEN.vi" "y_mobileye"(w627) -> ()
    }
    frame #2 {
      n476 = while {
        stop <- FALSE stop-if-true
        n477 = flat-sequence {
          frame #0 {
            n478 = Wait Until Next ms Multiple(millisecond multiple=u32 20 ("milliseconds to wait")) -> (millisecond timer value=w643:u32)
            n479 = feedback #5() -> (w645:u32)  [unwired: 1 in]
            n480 = feedback-in #5(w643) -> ()
            n481 = Subtract(x=w643, y=w645) -> (x-y=→"timmer 2":u32)
          }
          frame #1 {
            n482 = case shown="False" "Make WPT" {
              frame False {
                n483 = case shown="False" "Load WPT" {
                  frame False {
                    n484 = flat-sequence {
                      tunnel: [w654] -> w649
                      tunnel: w649 -> [w896]
                      frame #0 {
                        n485 = Select(t=9 ("Mission"), s=FALSE ("Parking mode"), f=0 ("Mission")) -> (s? t:f=w650:i32)
                        n486 = global write "G_PATH.vi" "Mission"(w650) -> ()
                      }
                      frame #1 {
                        n487 = disable-structure shown="Enabled" {
                          disable-tunnel: [_ w843] -> w654
                          frame Enabled {
                            n488 = flat-sequence {
                              tunnel: [w666] -> w656
                              tunnel: [w665] -> w655
                              tunnel: w656 -> [w823]
                              tunnel: w655 -> [w806]
                              frame #0 {
                                n489 = case shown="True" "mobileye" {
                                tunnel: [w681 w684] -> w660
                                frame False {
                                n490 = global write "G_SEN.vi" "lane_m_R"(1.75 ("lane_m_R")) -> ()
                                n491 = global write "G_SEN.vi" "lane_m_L"(-1.75 ("lane_m_L")) -> ()
                                n492 = local write "x"(0.0 ("x")) -> ()
                                n493 = Multiply(x="x", y=10.0) -> (x*y=w681:dbl)
                                }
                                frame True {
                                n494 = flat-sequence {
                                tunnel: [w796] -> w684
                                frame #0 {
                                n495 = global read "G_SEN.vi" "Lane_R_M"() -> (w691:dbl[])
                                n496 = global read "G_SEN.vi" "Lane_L_M"() -> (w698:dbl[])
                                n497 = Index Array(array=w691, index #1=0 ("index"), index #2=3 ("index")) -> (element #1=w690:dbl, element #2=w694:dbl)
                                n498 = Index Array(array=w698, index #1=0 ("index"), index #2=3 ("index")) -> (element #1=w686:dbl, element #2=w695:dbl)
                                n499 = Equal?(x=1.0, y=w690) -> (x = y?=w688:bool)
                                n500 = Equal?(x=1.0, y=w686) -> (x = y?=w685:bool)
                                n501 = case shown="True" w688 {
                                tunnel: w694 -> [_ w699]
                                frame False {
                                }
                                frame True {
                                n502 = flat-sequence {
                                tunnel: w699 -> [w705]
                                frame #0 {
                                w701 = 0.5 ("y")
                                n503 = global read "G_SEN.vi" "lane_m_R"() -> (w706:dbl)
                                n504 = Decrement(x=w701) -> (x-1=w700:dbl)
                                n505 = Multiply(x=w706, y=w701) -> (x*y=w704:dbl)
                                n506 = Multiply(x=w700, y=w705) -> (x*y=w703:dbl)
                                n507 = Subtract(x=w704, y=w703) -> (x-y=w702:dbl)
                                n508 = global write "G_SEN.vi" "lane_m_R"(w702) -> ()
                                }
                                frame #1 {
                                n509 = global read "G_SEN.vi" "Lane_L_M"() -> (w709:dbl[])
                                n510 = Index Array(array=w709, index=0) -> (element=w708:dbl)
                                n511 = Equal To 0?(x=w708) -> (x = 0?=w707:bool)
                                n512 = case shown="True" w707 {
                                frame False {
                                n513 = global read "G_SEN.vi" "Lane_L_M"() -> (w712:dbl[])
                                n514 = Index Array(array=w712, index #1=0 ("index"), index #2=3 ("index")) -> (element #1=w713:dbl, element #2=w717:dbl)
                                n515 = Not Equal?(x=w713, y=1.0) -> (x != y?=w715:bool)
                                n516 = case shown="True" w715 {
                                tunnel: w717 -> [_ w722]
                                frame False {
                                }
                                frame True {
                                n517 = global read "G_SEN.vi" "lane_m_R"() -> (w720:dbl)
                                n518 = Subtract(x=w720, y=3.3) -> (x-y=w721:dbl)
                                n519 = Max & Min(x=w722, y=w721) -> (max(x,y)=w718:dbl)  [unwired: 1 out]
                                n520 = global write "G_SEN.vi" "lane_m_L"(w718) -> ()
                                }
                                }
                                }
                                frame True {
                                n521 = global read "G_SEN.vi" "lane_m_R"() -> (w725:dbl)
                                n522 = Subtract(x=w725, y=3.3) -> (x-y=w723:dbl)
                                n523 = global write "G_SEN.vi" "lane_m_L"(w723) -> ()
                                }
                                }
                                }
                                }
                                }
                                }
                                n524 = case shown="True" w685 {
                                tunnel: w695 -> [_ w726]
                                frame False {
                                }
                                frame True {
                                n525 = flat-sequence {
                                tunnel: w726 -> [w732]
                                frame #0 {
                                w728 = 0.5 ("y")
                                n526 = global read "G_SEN.vi" "lane_m_L"() -> (w733:dbl)
                                n527 = Decrement(x=w728) -> (x-1=w727:dbl)
                                n528 = Multiply(x=w733, y=w728) -> (x*y=w731:dbl)
                                n529 = Multiply(x=w727, y=w732) -> (x*y=w730:dbl)
                                n530 = Subtract(x=w731, y=w730) -> (x-y=w729:dbl)
                                n531 = global write "G_SEN.vi" "lane_m_L"(w729) -> ()
                                }
                                frame #1 {
                                n532 = global read "G_SEN.vi" "Lane_R_M"() -> (w737:dbl[])
                                n533 = Index Array(array=w737, index=0) -> (element=w735:dbl)
                                n534 = Equal To 0?(x=w735) -> (x = 0?=w734:bool)
                                n535 = case shown="False" w734 {
                                frame False {
                                n536 = global read "G_SEN.vi" "Lane_R_M"() -> (w743:dbl[])
                                n537 = Index Array(array=w743, index #1=0 ("index"), index #2=3 ("index")) -> (element #1=w742:dbl, element #2=w738:dbl)
                                n538 = Not Equal?(x=w742, y=1.0) -> (x != y?=w740:bool)
                                n539 = case shown="True" w740 {
                                tunnel: w738 -> [_ w747]
                                frame False {
                                }
                                frame True {
                                n540 = global read "G_SEN.vi" "lane_m_L"() -> (w748:dbl)
                                n541 = Add(x=3.3 ("y"), y=w748) -> (x+y=w746:dbl)
                                n542 = Max & Min(x=w747, y=w746) -> (min(x,y)=w745:dbl)  [unwired: 1 out]
                                n543 = global write "G_SEN.vi" "lane_m_R"(w745) -> ()
                                }
                                }
                                }
                                frame True {
                                n544 = global read "G_SEN.vi" "lane_m_L"() -> (w750:dbl)
                                n545 = Add(x=3.3 ("y"), y=w750) -> (x+y=w752:dbl)
                                n546 = global write "G_SEN.vi" "lane_m_R"(w752) -> ()
                                }
                                }
                                }
                                }
                                }
                                }
                                }
                                frame #1 {
                                w758 = 0.8 ("y")
                                n547 = global read "G_SEN.vi" "Lane_R_M"() -> (w753:dbl[])
                                n548 = global read "G_SEN.vi" "Lane_L_M"() -> (w756:dbl[])
                                n549 = Index Array(array=w753, index=0) -> (element=w757:dbl)
                                n550 = Index Array(array=w756, index=0) -> (element=w759:dbl)
                                n551 = Equal?(x=w757, y=w758) -> (x = y?=w760:bool)
                                n552 = Equal?(x=w758, y=w759) -> (x = y?=w761:bool)
                                n553 = And(x=w760, y=w761) -> (x .and. y?=w762:bool)
                                n554 = case shown="True" w762 {
                                frame False {
                                }
                                frame True {
                                n555 = global read "G_SEN.vi" "Lane_R_M"() -> (w779:dbl[])
                                n556 = global read "G_SEN.vi" "Lane_L_M"() -> (w764:dbl[])
                                n557 = global read "G_SEN.vi" "lane_m_R"() -> (w772:dbl)
                                n558 = global read "G_SEN.vi" "lane_m_L"() -> (w771:dbl)
                                n559 = Index Array(array=w779, index=3) -> (element=w773:dbl)
                                n560 = Index Array(array=w764, index=3) -> (element=w770:dbl)
                                n561 = Subtract(x=w773, y=w772) -> (x-y=w778:dbl)
                                n562 = Subtract(x=w770, y=w771) -> (x-y=w765:dbl)
                                n563 = Absolute Value(x=w778) -> (abs(x)=w777:dbl)
                                n564 = Absolute Value(x=w765) -> (abs(x)=w766:dbl)
                                n565 = Less?(x=w777, y=1.5) -> (x < y?=w775:bool)
                                n566 = Less?(x=w766, y=1.5) -> (x < y?=w768:bool)
                                n567 = Select(t=w773, s=w775, f=w772) -> (s? t:f=w774:dbl)
                                n568 = Select(t=w770, s=w768, f=w771) -> (s? t:f=w769:dbl)
                                n569 = global write "G_SEN.vi" "lane_m_R"(w774) -> ()
                                n570 = global write "G_SEN.vi" "lane_m_L"(w769) -> ()
                                }
                                }
                                }
                                frame #2 {
                                w793 = 0.05 ("y")
                                n571 = global read "G_SEN.vi" "lane_m_L"() -> (w799:dbl)
                                n572 = global read "G_SEN.vi" "lane_m_R"() -> (w798:dbl)
                                n573 = Add(x=w799, y=w798) -> (x+y=w795:dbl)
                                n574 = local read "x"() -> (w783:dbl)
                                n575 = Multiply(x=w795, y=0.5) -> (x*y=w782:dbl)
                                n576 = Subtract(x=w783, y=w782) -> (x-y=w788:dbl)
                                n577 = Absolute Value(x=w788) -> (abs(x)=w787:dbl)
                                n578 = Decrement(x=w793) -> (x-1=w792:dbl)
                                n579 = Greater?(x=w787, y=0.95) -> (0:w785:bool)
                                n580 = Select(t=w783, s=w785, f=w782) -> (s? t:f=w784:dbl)
                                n581 = local read "x"() -> (w781:dbl)
                                n582 = Multiply(x=w792, y=w781) -> (x*y=w791:dbl)
                                n583 = Multiply(x=w784, y=w793) -> (x*y=w790:dbl)
                                n584 = Subtract(x=w790, y=w791) -> (x-y=w789:dbl)
                                n585 = local write "x"(w789) -> ()
                                n586 = Multiply(x=w789, y=10.0) -> (x*y=w796:dbl)
                                }
                                }
                                }
                                }
                                n587 = flat-sequence {
                                tunnel: [w668] -> w657
                                frame #0 {
                                n588 = global read "G_NAV.vi" "M6006"() -> (w677:T7)
                                n589 = Unbundle By Name(w677) -> ("lcc[1]"=w673:dbl, "lcc[0]"=w672:dbl, "attitude[2]"=w671:dbl)
                                n590 = global read "G_VEH.vi" "xyhc"() -> (w676:T4)
                                n591 = Unbundle By Name(w676) -> ("x"=w675:dbl, "y"=w674:dbl)
                                n592 = Negate(x=w671) -> (-x=w670:dbl)
                                n593 = call "rotm_siso.vi"("angle[rad]"=w670, "y0"=w672, "x0"=w673, "y"=w674, "x"=w675) -> ("x'"=w667:dbl)  [unwired: 5 in, 1 out]
                                n594 = Multiply(x=w667, y=-10.0) -> (x*y=w668:dbl)
                                }
                                }
                                n595 = Add(x="x 2", y=w660) -> (x+y=w659:dbl)
                                n596 = Add(x=w659, y=w657) -> (x+y=w658:dbl)
                                n597 = Multiply(x=w659, y=0.1) -> (x*y=w665:dbl)
                                n598 = call "pathtracking.vi"("x"=w658, "y"="y") -> ("R"=w666:dbl)  [unwired: 9 in]
                              }
                              frame #1 {
                                w833 = 0.04 ("y")
                                n599 = global read "G_VEH.vi" "C_Wheel base"() -> (w841:dbl)
                                n600 = Divide(x=w841, y=w823) -> (x/y=w840:dbl)
                                n601 = global read "G_VEH.vi" "candata"() -> (w811:T8)
                                n602 = Inverse Tangent(1:w840) -> (0:w839:dbl)
                                n603 = Unbundle By Name(w811) -> ("VS_can"=w804:dbl)
                                n604 = Divide(x=w806, y=-12.0) -> (x/y=w826:dbl)
                                n605 = Multiply(x=w839, y=180.0) -> (x*y=w837:dbl)
                                n606 = global read "G_VEH.vi" "ratio_steer"() -> (w834:dbl)
                                n607 = global read "G_VEH.vi" "candata"() -> (w842:T8)
                                n608 = Divide(x=w837, y=3.141592653589793) -> (x/y=w835:dbl)
                                n609 = Divide(x=w804, y=3.6) -> (x/y=w803:dbl)
                                n610 = In Range and Coerce(upper limit=1.0, x=w826, lower limit=-1.0) -> (coerced(x)=w813:dbl)  [unwired: 1 out]
                                n611 = Unbundle By Name(w842) -> ("Steer_output"=w828:dbl)
                                n612 = Multiply(x=w835, y=w834) -> (x*y=w827:dbl)
                                n613 = Absolute Value(x=w803) -> (abs(x)=w810:dbl)
                                n614 = Decrement(x=w833) -> (x-1=w832:dbl)
                                n615 = Multiply(x=w827, y=w833) -> (x*y=w830:dbl)
                                n616 = feedback #6(w828) -> (w831:dbl)
                                n617 = Multiply(x=w832, y=w831) -> (x*y=w829:dbl)
                                n618 = Increment(x=w810) -> (x+1=w808:dbl)
                                n619 = Multiply(x=500.0, y=w813) -> (x*y=w809:dbl)
                                n620 = Divide(x=w809, y=w808) -> (x/y=w801:dbl)
                                n621 = Subtract(x=w830, y=w829) -> (x-y=w800:dbl)
                                n622 = feedback-in #6(w800) -> ()
                                n623 = global read "G_VEH.vi" "ratio_steer"() -> (w822:dbl)
                                n624 = Add(x=w801, y=w800) -> (x+y=w807:dbl)
                                n625 = Divide(x=w807, y=w822) -> (x/y=w821:dbl)
                                n626 = global write "G_VEH.vi" "handle"(w807) -> ()
                                n627 = Multiply(x=3.141592653589793, y=w821) -> (x*y=w819:dbl)
                                n628 = global read "G_VEH.vi" "C_Wheel base"() -> (w816:dbl)
                                n629 = Divide(x=w819, y=180.0) -> (x/y=w817:dbl)
                                n630 = Tangent(1:w817) -> (0:w815:dbl)
                                n631 = Divide(x=w816, y=w815) -> (x/y=w814:dbl)
                                n632 = global write "G_VEH.vi" "Rtmp"(w814) -> ()
                              }
                            }
                          }
                          frame Disabled {
                            n633 = flat-sequence {
                              tunnel: [w880] -> w849
                              frame #0 {
                                n634 = global read "G_VEH.vi" "candata"() -> (w879:T8)
                                n635 = Unbundle By Name(w879) -> ("VS_can"=w878:dbl)
                                n636 = Multiply(x=w878, y=0.5) -> (x*y=w876:dbl)
                                n637 = In Range and Coerce(upper limit=50.0, x=w876, lower limit=40.0) -> (coerced(x)=w873:dbl)  [unwired: 1 out]
                                n638 = Multiply(x=w873, y=w873) -> (x*y=w884:dbl)
                                n639 = Multiply(x=w873, y=w884) -> (x*y=w886:dbl)
                                n640 = Multiply(x=w884, y=0.5) -> (x*y=w881:dbl)
                                n641 = Divide(x=w886, y=3.0) -> (x/y=w882:dbl)
                                n642 = Build Array(w882, w881, w873) -> (w880:dbl[])
                              }
                            }
                            n643 = flat-sequence {
                              tunnel: [w864] -> w857
                              tunnel: [w859] -> w843
                              frame #0 {
                                n644 = global read "G_SEN.vi" "Lane_R_M"() -> (w867:dbl[])
                                n645 = global read "G_SEN.vi" "Lane_L_M"() -> (w868:dbl[])
                                n646 = Multiply(x=w868, y=0.5) -> (x*y=w871:dbl[])
                                n647 = Multiply(x=w867, y=0.5) -> (x*y=w872:dbl[])
                                n648 = Add(x=w871, y=w872) -> (x+y=w863:dbl[])
                                n649 = global write "G_SEN.vi" "Lane_C_I"(w863) -> ()
                                n650 = Index Array(array=w863, index=0) -> (element=w861:dbl)
                                n651 = Array Subset(array=w863, index=1, length=3) -> (w864:dbl[])
                                n652 = Less?(x=w861, y=0.8) -> (x < y?=w859:bool)
                              }
                            }
                            n653 = Multiply(x=w857, y=w849) -> (x*y=w858:dbl[])
                            n654 = Add Array Elements(numeric array=w858) -> (sum=w848:dbl)
                            n655 = global read "G_VEH.vi" "candata"() -> (w845:T8)
                            n656 = Select(t=0.0, s=w843, f=w848) -> (s? t:f=w847:dbl)
                            n657 = Unbundle By Name(w845) -> ("Steer_output"=w844:dbl)
                            n658 = Multiply(x=-0.2, y=w847) -> (x*y=w855:dbl)
                            n659 = Multiply(x=w855, y=0.1 ("x")) -> (x*y=w853:dbl)
                            n660 = Multiply(x=0.9, y=w844) -> (x*y=w852:dbl)
                            n661 = Add(x=w853, y=w852) -> (x+y=w851:dbl)
                          }
                        }
                      }
                      frame #2 {
                        n662 = global read "G_VEH.vi" "candata"() -> (w895:T8)
                        n663 = Unbundle By Name(w895) -> ("VS_can"=w894:dbl)
                        n664 = Multiply(x=w894, y=0.9) -> (x*y=w892:dbl)
                        n665 = Max & Min(x=10.0, y=w892) -> (max(x,y)=w889:dbl)  [unwired: 1 out]
                        n666 = Max & Min(x=w889, y="Max. Vel.") -> (min(x,y)=w887:dbl)  [unwired: 1 out]
                        n667 = Select(t=w887, s=w896, f="Max. Vel.") -> (s? t:f=w890:dbl)
                        n668 = call "collision_fixed_steer.vi"("obsclose"="obs", "Max. Vel."=w890) -> ("collision"=w898:bool, "speed limit"=→"Speed limit":dbl)  [unwired: 8 in]
                        "collision" <- w898
                        n669 = Boolean To (0,1)(Boolean=w898) -> (0, 1=→"col":i16)
                      }
                      frame #3 {
                        n670 = global read "G_PATH.vi" "Mission"() -> (w901:i32)
                        "Mission" <- w901
                        n671 = case shown="9" w901 {
                          frame 0, Default {
                          }
                          frame 9 {
                            n672 = flat-sequence {
                              frame #0 {
                                n673 = global write "G_PATH.vi" "parking_cost"(0 ("parkingcost")) -> ()
                                n674 = global write "G_VEH.vi" "xparking"(T14 {"c_idx"=-1, "xc"=0.0, "yc"=0.0, "hc"=0.0, "xc_path"=0.0} ("xparking")) -> ()
                                n675 = global write "G_PATH.vi" "wpt_park"(dbl[][] [] ("wpt_park")) -> ()
                              }
                              frame #1 {
                                n676 = global read "G_PATH.vi" "path_rev"() -> (w905:dbl[][])
                                n677 = Empty Array?(array=w905) -> (empty?=w906:bool)
                                n678 = case shown="False" w906 {
                                frame False {
                                n679 = flat-sequence {
                                frame #0 {
                                n680 = disable-structure shown="Enabled" {
                                frame Enabled {
                                n681 = global read "G_PATH.vi" "path_rev"() -> (w912:dbl[][])
                                n682 = global read "G_VEH.vi" "xyhp"() -> (w907:T4)
                                n683 = Empty Array?(array=w912) -> (empty?=w911:bool)
                                n684 = Unbundle By Name(w907) -> ("idx"=w913:i32)
                                n685 = Not(x=w911) -> (.not. x?=w910:bool)
                                n686 = Equal To 0?(x=w913) -> (x = 0?=w909:bool)
                                n687 = And(x=w910, y=w909) -> (x .and. y?=w908:bool)
                                n688 = case shown="True" w908 {
                                frame False {
                                }
                                frame True {
                                n689 = flat-sequence {
                                tunnel: [w917] -> w914
                                frame #0 {
                                n690 = global read "G_PATH.vi" "path_rev"() -> (w915:dbl[][])
                                n691 = global write "G_PATH.vi" "path"(w915) -> ()
                                n692 = global write "G_PATH.vi" "path_origin"(w915) -> ()
                                }
                                frame #1 {
                                n693 = call "whereami.vi"() -> ()  [unwired: 12 in]
                                }
                                frame #2 {
                                n694 = global read "G_PATH.vi" "path"() -> (w916:dbl[][])
                                n695 = global read "G_VEH.vi" "xyhc"() -> (w918:T4)
                                n696 = call "findcurrentpointinpath.vi"("xyhc_in"=w918, "path_updated"=w916) -> ("xyhc_out"=w917:T4)  [unwired: 8 in, 1 out]
                                }
                                }
                                n697 = global write "G_VEH.vi" "xyhc"(w914) -> ()
                                }
                                }
                                }
                                frame Disabled {
                                }
                                }
                                }
                                frame #1 {
                                n698 = global read "G_VEH.vi" "xparking"() -> (w939:T4)
                                n699 = global read "G_NAV.vi" "M6006"() -> (w938:T7)
                                n700 = Unbundle By Name(w938) -> ("lcc[1]"=w936:dbl, "lcc[0]"=w934:dbl)
                                n701 = Unbundle By Name(w939) -> ("x"=w937:dbl, "y"=w935:dbl)
                                n702 = Subtract(x=w937, y=w936) -> (x-y=w933:dbl)
                                n703 = Subtract(x=w935, y=w934) -> (x-y=w932:dbl)
                                n704 = global read "G_VEH.vi" "candata"() -> (w926:T8)
                                n705 = Square(x=w933) -> (x^2=w931:dbl)
                                n706 = Square(x=w932) -> (x^2=w930:dbl)
                                n707 = Unbundle By Name(w926) -> ("VS_can"=w925:dbl)
                                n708 = Add(x=w931, y=w930) -> (x+y=w929:dbl)
                                n709 = Absolute Value(x=w925) -> (abs(x)=w924:dbl)
                                n710 = Square Root(x=w929) -> (sqrt(x)=w928:dbl)
                                n711 = global read "G_VEH.vi" "firstcall"() -> (w919:bool)
                                n712 = Less?(x=w928, y=1.2) -> (x < y?=w922:bool)
                                n713 = Less?(x=w924, y=0.05) -> (x < y?=w921:bool)
                                n714 = Compound Arithmetic op=AND(w919, w922, w921) -> (w920:bool)
                                n715 = case shown="False" w920 {
                                tunnel: w928 -> [w940 _]
                                frame False {
                                n716 = global read "G_SEN.vi" "sensor_etc"() -> (w943:dbl[][])
                                n717 = global read "G_VEH.vi" "candata"() -> (w950:T8)
                                n718 = Unbundle By Name(w950) -> ("VS_can"=w949:dbl)
                                n719 = Empty Array?(array=w943) -> (empty?=w942:bool)
                                n720 = In Range and Coerce(upper limit=6.0, x=w940, lower limit=1.5) -> (In Range?=w948:bool)  [unwired: 1 out]
                                n721 = Less Or Equal To 0?(x=w949) -> (x <= 0?=w947:bool)
                                n722 = Not(x=w942) -> (.not. x?=w941:bool)
                                n723 = Compound Arithmetic op=AND(w947, w948, w941) -> (w946:bool)
                                n724 = case shown="True" w946 {
                                frame False {
                                }
                                frame True {
                                n725 = global write "G_VEH.vi" "firstcall"(TRUE ("firstcall")) -> ()
                                n726 = call "parking_ung2rev.vi"() -> ()  [unwired: 12 in]
                                }
                                }
                                }
                                frame True {
                                n727 = flat-sequence {
                                frame #0 {
                                n728 = global write "G_VEH.vi" "firstcall"(FALSE ("firstcall")) -> ()
                                n729 = global write "G_VEH.vi" "parking_loop"(TRUE ("parking_loop")) -> ()
                                }
                                frame #1 {
                                n730 = call "parking_ung2_loop.vi"() -> ()  [unwired: 12 in]
                                }
                                }
                                }
                                }
                                }
                                }
                                }
                                frame True {
                                n731 = global read "G_VEH.vi" "xmission"() -> (w967:T4)
                                n732 = global read "G_NAV.vi" "M6006"() -> (w966:T7)
                                n733 = global write "G_VEH.vi" "parking_loop"(FALSE ("parking_loop")) -> ()
                                n734 = global write "G_VEH.vi" "firstcall"(TRUE ("firstcall")) -> ()
                                n735 = Unbundle By Name(w966) -> ("lcc[1]"=w964:dbl, "lcc[0]"=w962:dbl)
                                n736 = Unbundle By Name(w967) -> ("x"=w965:dbl, "y"=w963:dbl)
                                n737 = Subtract(x=w965, y=w964) -> (x-y=w961:dbl)
                                n738 = Subtract(x=w963, y=w962) -> (x-y=w960:dbl)
                                n739 = Square(x=w961) -> (x^2=w959:dbl)
                                n740 = Square(x=w960) -> (x^2=w958:dbl)
                                n741 = Add(x=w959, y=w958) -> (x+y=w957:dbl)
                                n742 = Square Root(x=w957) -> (sqrt(x)=w956:dbl)
                                n743 = Greater?(x=w956, y=5.0) -> (0:w954:bool)
                                n744 = case shown="True" w954 {
                                frame False {
                                }
                                frame True {
                                n745 = call "parking_ung2.vi"() -> ()  [unwired: 12 in]
                                }
                                }
                                }
                                }
                              }
                            }
                          }
                        }
                      }
                    }
                  }
                  frame True {
                    n746 = flat-sequence {
                      frame #0 {
                        w971 = FALSE ("X Scale.Loose Fit")
                        w970 = u8 0 ("X Scale.Scale Fit")
                        n747 = call "initvar.vi"() -> ()  [unwired: 12 in]
                        n748 = property on="XY Graph" class="XYGraph (strict)"("XScale.ScaleFit"=w970, "YScale.ScaleFit"=w970, "XScale.LooseFit"=w971, "YScale.LooseFit"=w971) -> ()  [unwired: 2 in, 2 out]
                      }
                      frame #1 {
                        n749 = global read "G_VEH.vi" "Location"() -> (w972:i32)
                        n750 = Bundle("Minimum"=-22.6, "Minimum"=22.6, "Minimum"=10.0, "Minimum"=1.0, "Minimum"=-20.0) -> (w985:T15)  [unwired: 1 in]
                        n751 = Bundle("Minimum"=-5.0, "Minimum"=37.3, "Minimum"=10.0, "Minimum"=1.0, "Minimum"=-20.0) -> (w978:T15)  [unwired: 1 in]
                        n752 = property on="XY Graph" class="XYGraph (strict)"("XScale.Range"=w985) -> ()  [unwired: 2 in, 2 out]
                        n753 = property on="XY Graph" class="XYGraph (strict)"("YScale.Range"=w978) -> ()  [unwired: 2 in, 2 out]
                        n754 = call "getecefdcmref.vi"("map"=w972) -> ("XYZ"=w973:dbl[])  [unwired: 10 in, 4 out]
                        n755 = global write "G_NAV.vi" "ecef ref"(w973) -> ()
                      }
                      frame #2 {
                        n756 = global read "G_DATA.vi" "path"() -> (w988:path)
                        n757 = Build Path(base path=w988, name or relative path="wpt") -> (appended path=w986:path)
                        n758 = call "Read From Measurement File2"("Filename"=w986, "Reset"=TRUE) -> ("error out"=w990:errorcluster, "Signals"=w992:dynamicdata)  [unwired: 4 in, 4 out]
                        n759 = Unbundle By Name(w990) -> ("status"=w989:bool)
                        n760 = case shown="False" w989 {
                          tunnel: w992 -> [w993 _]
                          frame False {
                            n761 = call "Convert from Dynamic Data2"("Dynamic Data Type"=w993) -> ("Array"=w995:dbl[][])  [unwired: 3 in]
                            n762 = Empty Array?(array=w995) -> (empty?=w994:bool)
                            n763 = case shown="False" w994 {
                              tunnel: w995 -> [w996 _]
                              frame False {
                                n764 = call "path_ini_new.vi"("WPT"=w996) -> ()  [unwired: 11 in]
                              }
                              frame True {
                                w997 = T16 [] ("Missions_origin")
                                w998 = dbl[][] [] ("path_updated")
                                n765 = global write "G_PATH.vi" "path"(w998) -> ()
                                n766 = global write "G_PATH.vi" "path_very_origin"(w998) -> ()
                                n767 = global write "G_PATH.vi" "path_origin"(w998) -> ()
                                n768 = global write "G_PATH.vi" "Missions_origin"(w997) -> ()
                                n769 = global write "G_PATH.vi" "Missions"(w997) -> ()
                              }
                            }
                          }
                          frame True {
                          }
                        }
                      }
                      frame #3 {
                        n770 = disable-structure shown="Enabled" {
                          disable-tunnel: [w1000 _] -> w999
                          frame Disabled {
                            n771 = disable-structure shown="Enabled" {
                              disable-tunnel: [w1006 _] -> w1003
                              disable-tunnel: [w1004 errorcluster {"status"=TRUE, "code"=0, "source"=""} ("error out")] -> w1002
                              frame Enabled {
                                n772 = call "Read From Measurement File"("Reset"=TRUE) -> ("error out"=w1004:errorcluster, "Signals"=w1006:dynamicdata)  [unwired: 5 in, 4 out]
                              }
                              frame Disabled {
                              }
                            }
                            n773 = Unbundle By Name(w1002) -> ("status"=w1001:bool)
                            n774 = case shown="False" w1001 {
                              tunnel: w1003 -> [w1012 _]
                              tunnel: [w1008 _] -> w1000
                              frame False {
                                n775 = call "Convert from Dynamic Data"("Dynamic Data Type"=w1012) -> ("Array"=w1009:dbl[][])  [unwired: 3 in]
                                n776 = for {
                                tunnel: w1009 -> [w1020] mode=indexing
                                tunnel: [w1014] -> w1010 mode=indexing
                                w1013 = T4 {"idx"=0, "x"=0.0, "y"=0.0, "h"=0.0, "x_path"=0.0}  # x
                                n777 = Index Array(array=w1020, index #1=0 ("index")) -> (element #1=w1018:dbl, element #2=w1017:dbl, element #3=w1016:dbl)  [unwired: 2 in]
                                n778 = Bundle By Name(cluster=w1013, "idx"=w1018, "x"=w1017, "y"=w1016) -> (w1015:T4)
                                n779 = Build Cluster Array(w1015) -> (w1014:T17)
                                }
                                n780 = Index Array(array=w1010, index (col)=0 ("disabled index (col)")) -> (element=w1008:T17)  [unwired: 1 in]
                              }
                              frame True {
                              }
                            }
                          }
                          frame Enabled {
                          }
                        }
                        n781 = global write "G_PATH.vi" "Missions_origin"(w999) -> ()
                        n782 = global write "G_PATH.vi" "Missions"(w999) -> ()
                      }
                      frame #4 {
                        n783 = global read "G_VEH.vi" "Location"() -> (w1021:i32)
                        n784 = local write "Load WPT"(FALSE ("Load WPT")) -> ()
                        n785 = call "mapconf.vi"("Location"=w1021) -> ("y"=w1023:cluster{dbl, dbl, "y":dbl, "y":dbl, dbl}, "x"=w1024:cluster{dbl, dbl, "y":dbl, "y":dbl, dbl}, "new picture"=w1025:picture)  [unwired: 8 in]
                        n786 = property on="XY Graph 2" class="XYGraph (strict)"("PlotImages.Back"=w1025) -> ()  [unwired: 2 in, 2 out]
                        n787 = property on="XY Graph 2" class="XYGraph (strict)"("XScale.Range"=w1024, "YScale.Range"=w1023) -> ()  [unwired: 2 in, 2 out]
                      }
                    }
                  }
                }
              }
              frame True {
                n788 = flat-sequence {
                  tunnel: [w1032] -> w1026
                  tunnel: w1026 -> [w1121]
                  frame #0 {
                    w1027 = 0.0
                    n789 = disable-structure shown="Enabled" {
                      frame Disabled {
                        w1028 = TRUE ("X Scale.Loose Fit")
                        w1029 = u8 2 ("X Scale.Scale Fit")
                        n790 = property on="XY Graph" class="XYGraph (strict)"("XScale.ScaleFit"=w1029, "YScale.ScaleFit"=w1029, "XScale.LooseFit"=w1028, "YScale.LooseFit"=w1028) -> ()  [unwired: 2 in, 2 out]
                      }
                      frame Enabled {
                      }
                    }
                    n791 = global write "G_VEH.vi" "handle"(w1027) -> ()
                    n792 = global write "G_VEH.vi" "VS_des"(w1027) -> ()
                  }
                  frame #1 {
                    n793 = local read "Make WPT"() -> (w1031:bool)
                    n794 = global read "G_VEH.vi" "Location"() -> (w1030:i32)
                    n795 = Initialize Array(0.0 ("element"), 7 ("dimension size"), 1 ("dimension size")) -> (w1033:dbl[][])
                    n796 = while {
                      shift-right: [w1038] -> w1032
                      shift-left: w1033 -> [w1040]
                      shift-right: [FALSE] -> _
                      shift-left: w1031 -> [w1041]
                      tunnel: w1030 -> [w1037]
                      stop <- w1043 stop-if-true
                      n797 = local read "Make WPT"() -> (w1044:bool)
                      n798 = flat-sequence {
                        tunnel: [w1053] -> w1039
                        tunnel: w1037 -> [w1046]
                        frame #0 {
                          n799 = global read "G_NAV.vi" "GPS_status"() -> (w1045:T18)
                          n800 = disable-structure shown="Enabled" {
                            disable-tunnel: [w1064 w1068] -> w1056
                            disable-tunnel: [w1063 w1067] -> w1055
                            disable-tunnel: [w1057 w1066] -> w1054
                            disable-tunnel: w1045 -> [w1062 w1076]
                            disable-tunnel: [w1061 w1075] -> w1052
                            disable-tunnel: [w1060 w1074] -> w1051
                            disable-tunnel: [w1057 w1073] -> w1050
                            disable-tunnel: w1046 -> [_ w1072]
                            frame Enabled {
                              n801 = global read "G_NAV.vi" "M6006"() -> (w1065:T7)
                              n802 = Unbundle By Name(w1065) -> ("lcc[0]"=w1059:dbl, "lcc[1]"=w1058:dbl)
                              n803 = Unbundle By Name(w1062) -> ("lat"=w1061:dbl, "lon"=w1060:dbl, "hgt"=w1057:dbl)
                              n804 = To Double Precision Float(number=w1059) -> (double precision float=w1064:dbl)
                              n805 = To Double Precision Float(number=w1058) -> (double precision float=w1063:dbl)
                            }
                            frame Disabled {
                              n806 = Unbundle By Name(w1076) -> ("lat"=w1075:dbl, "lon"=w1074:dbl, "hgt"=w1073:dbl)
                              n807 = call "getecefdcmref.vi"("map"=w1072) -> ("XYZ"=w1071:dbl[])  [unwired: 10 in, 4 out]
                              n808 = call "llh2lcc.vi"("ecef ref"=w1071, "hgt"=w1073, "lon"=w1074, "lat"=w1075) -> ("lcc"=w1070:dbl[])  [unwired: 7 in]
                              n809 = Index Array(array=w1070, index #1=0 ("index")) -> (element #1=w1068:dbl, element #2=w1067:dbl, element #3=w1066:dbl)  [unwired: 2 in]
                            }
                          }
                          n810 = global read "G_VEH.vi" "candata"() -> (w1049:T8)
                          n811 = Unbundle By Name(w1049) -> ("VS_can"=w1048:dbl)
                          n812 = To Double Precision Float(number=w1046) -> (double precision float=w1047:dbl)
                          n813 = Build Array(w1052, w1051, w1050, w1056, w1055, w1054, w1048, w1047) -> (w1053:dbl[])
                        }
                      }
                      n814 = Not(x=w1044) -> (.not. x?=w1043:bool)
                      n815 = case shown="False" w1041 {
                        tunnel: w1040 -> [w1091 w1108]
                        tunnel: w1039 -> [w1090 w1106]
                        tunnel: [w1089 w1105] -> w1038
                        frame False {
                          n816 = Array Size(array=w1091) -> (size(s)=w1099:i32[])
                          n817 = Index Array(array=w1099, index=1) -> (element=w1088:i32)
                          n818 = Decrement(x=w1088) -> (x-1=w1087:i32)
                          n819 = Index Array(array=w1091, index (col)=w1087) -> (element=w1095:dbl[])  [unwired: 1 in]
                          n820 = Index Array(array=w1095, index #1=3 ("index"), index #2=4 ("index")) -> (element #1=w1086:dbl, element #2=w1084:dbl)
                          n821 = Index Array(array=w1090, index #1=3 ("index"), index #2=4 ("index")) -> (element #1=w1085:dbl, element #2=w1083:dbl)
                          n822 = Subtract(x=w1086, y=w1085) -> (x-y=w1082:dbl)
                          n823 = Subtract(x=w1084, y=w1083) -> (x-y=w1081:dbl)
                          n824 = Square(x=w1082) -> (x^2=w1080:dbl)
                          n825 = Square(x=w1081) -> (x^2=w1079:dbl)
                          n826 = Add(x=w1080, y=w1079) -> (x+y=w1078:dbl)
                          n827 = Greater Or Equal?(x=w1078, y=0.25) -> (x >= y?=w1092:bool)
                          n828 = case shown="True" w1092 {
                            tunnel: w1091 -> [w1100 w1104]
                            tunnel: w1088 -> [_ w1101]
                            tunnel: w1090 -> [_ w1103]
                            tunnel: [w1100 w1102] -> w1089
                            frame False {
                            }
                            frame True {
                              n829 = Insert Into Array(array=w1104, index (col)=w1101, new element=w1103) -> (w1102:dbl[][])  [unwired: 1 in]
                            }
                          }
                        }
                        frame True {
                          n830 = Replace Array Subset(array=w1108, new element=w1106, index (col)=0 ("disabled index (col)")) -> (w1105:dbl[][])  [unwired: 1 in]
                        }
                      }
                    }
                  }
                  frame #2 {
                    n831 = call "Convert to Dynamic Data"("2D Array"=w1121) -> ("Dynamic Data Type"=w1122:dynamicdata)  [unwired: 3 in]
                    n832 = global read "G_VEH.vi" "Location"() -> (w1118:i32)
                    n833 = case shown="9" w1118 {
                      tunnel: ["" ("String") "Hyundai" ("String") "KAIST" ("String") "AJOU" ("String") "MUNJI" ("String") "Airforce" ("String") "CAR" ("String") "KATRI" ("String") _ "coex" ("String")] -> w1117
                      frame 0, Default {
                      }
                      frame 1 {
                      }
                      frame 2 {
                      }
                      frame 3 {
                      }
                      frame 4 {
                      }
                      frame 5 {
                      }
                      frame 6 {
                      }
                      frame 7 {
                      }
                      frame 8 {
                      }
                      frame 9 {
                      }
                    }
                    n834 = Get Date/Time In Seconds() -> (seconds since 1Jan1904=w1119:timestamp)
                    n835 = Format Date/Time String(time format string (%c)="%2y%2m%2d%2H%2M", seconds (now)=w1119) -> (date/time string=w1115:string)  [unwired: 1 in]
                    n836 = global read "G_DATA.vi" "path"() -> (w1113:path)
                    n837 = Build Path(base path=w1113, name or relative path="wpt") -> (appended path=w1111:path)
                    n838 = Concatenate Strings(w1115, "_" ("string"), w1117, ".lvm" ("string")) -> (w1110:string)
                    n839 = Build Path(base path=w1111, name or relative path=w1110) -> (appended path=w1109:path)
                    n840 = call "save wpt"("Signals"=w1122, "Reset"=TRUE, "Filename"=w1109) -> ()  [unwired: 14 in, 3 out]
                  }
                }
              }
            }
          }
        }
      }
    }
  }
